vi "Control_Sensing_Sep.vi"() -> ()   [LabVIEW 2019]
uses:
  Control 1.ctl
  <vilib>/myRIO/Instrument Drivers/Onboard IO/I2C/typedefs/I2C User Configuration.ctl
  <vilib>/myRIO/Instrument Drivers/Onboard IO/I2C/typedefs/I2C Transfer Rate.ctl
  <vilib>/myRIO/Instrument Drivers/Onboard IO/I2C/typedefs/I2C Reference.ctl
  <vilib>/myRIO/Common/Instrument Driver Framework/Utilities/typedefs/myRIO Generic Hardware Reference.ctl
  <vilib>/myRIO/Common/Instrument Driver Framework/Utilities/typedefs/Hardware Version Enum.ctl
  <vilib>/myRIO/Common/Instrument Driver Framework/Utilities/typedefs/myRIO v1.0 Reference.ctl
  <vilib>/myRIO/Common/Instrument Driver Framework/Utilities/typedefs/Generic FPGA Reference.ctl
  <vilib>/myRIO/Common/Instrument Driver Framework/myRIO v1.0/I2C/typedefs/I2C Channels Enum.ctl
  <vilib>/myRIO/Instrument Drivers/Onboard IO/I2C/typedefs/I2C Configuration.ctl
  <vilib>/userDefined/High Color/nirio_resource_hc.ctl
  <vilib>/myRIO/Instrument Drivers/Onboard IO/DIO/typedefs/DIO Reference.ctl
  <vilib>/myRIO/Common/Instrument Driver Framework/myRIO v1.0/DIO/typedefs/DIO Channels List.ctl
  <vilib>/myRIO/Common/Instrument Driver Framework/myRIO v1.0/DIO/typedefs/DIO Channels Enum.ctl
  <vilib>/myRIO/Instrument Drivers/Onboard IO/AI/typedefs/AI Reference.ctl
  <vilib>/myRIO/Common/Instrument Driver Framework/myRIO v1.0/AI/typedefs/AI Channels List.ctl
  <vilib>/myRIO/Common/Instrument Driver Framework/myRIO v1.0/AI/typedefs/AI Channels Enum.ctl
  <vilib>/myRIO/Common/Instrument Driver Framework/Utilities/typedefs/Analog Scaling Constants List.ctl
  <vilib>/myRIO/Common/Instrument Driver Framework/Utilities/typedefs/Analog Scaling Constants.ctl
  <vilib>/myRIO/Instrument Drivers/Onboard IO/PWM/typedefs/PWM Reference.ctl
  <vilib>/myRIO/Common/Instrument Driver Framework/myRIO v1.0/PWM/typedefs/PWM Channels Enum.ctl
  <vilib>/myRIO/Instrument Drivers/Onboard IO/PWM/typedefs/PWM Configuration.ctl
  <vilib>/myRIO/Common/Instrument Driver Framework/Utilities/vis/Is FPGA Ref Available.vi
  <vilib>/myRIO/Common/Instrument Driver Framework/myRIO v1.0/I2C/vis/myRIO v1.1 Open I2C.vi
  <vilib>/myRIO/Instrument Drivers/Onboard IO/I2C/vis/Configure.vi
  <vilib>/myRIO/Instrument Drivers/Onboard IO/I2C/vis/Write.vi
  <vilib>/myRIO/Common/Instrument Driver Framework/myRIO v1.0/DIO/vis/myRIO v1.1 Open DIO.vi
  <vilib>/myRIO/Instrument Drivers/Onboard IO/DIO/vis/Write.vi
  <vilib>/myRIO/Common/Instrument Driver Framework/myRIO v1.0/AI/vis/myRIO v1.1 Open AI.vi
  <vilib>/myRIO/Instrument Drivers/Onboard IO/AI/vis/Read.vi
  <vilib>/myRIO/Common/Instrument Driver Framework/myRIO v1.0/PWM/vis/myRIO v1.1 Open PWM.vi
  <vilib>/myRIO/Instrument Drivers/Onboard IO/PWM/vis/Set Duty Cycle and Frequency.vi
  <vilib>/myRIO/Instrument Drivers/Onboard IO/I2C/vis/Write Read.vi
  <vilib>/myRIO/Common/Instrument Driver Framework/myRIO v1.0/UART/vis/myRIO v1.0 Close UART.vi
  <vilib>/myRIO/Common/Instrument Driver Framework/Utilities/vis/Validate Channels.vi
  <vilib>/myRIO/Common/Instrument Driver Framework/myRIO v1.0/I2C/vis/myRIO v1.0 Reserve I2C.vi
  <vilib>/myRIO/Common/Instrument Driver Framework/myRIO v1.0/DIO/vis/myRIO v1.0 Reserve DIO.vi
  <vilib>/myRIO/Common/Instrument Driver Framework/myRIO v1.0/AI/vis/myRIO v1.0 Reserve AI.vi
  <vilib>/myRIO/Common/Instrument Driver Framework/myRIO v1.0/PWM/vis/myRIO v1.0 Reserve PWM.vi
  <vilib>/myRIO/Common/Instrument Driver Framework/myRIO v1.0/I2C/vis/myRIO v1.0 Build MUX Configuration I2C.vi
  <vilib>/myRIO/Common/Instrument Driver Framework/myRIO v1.0/Resource Manager/vis/myRIO v1.0 Reserve Channel List.vi
  <vilib>/myRIO/Common/Instrument Driver Framework/myRIO v1.0/DIO/vis/myRIO v1.0 Build MUX Configuration DIO.vi
  <vilib>/myRIO/Common/Instrument Driver Framework/myRIO v1.0/AI/vis/myRIO v1.0 Build MUX Configuration AI.vi
  <vilib>/myRIO/Common/Instrument Driver Framework/myRIO v1.0/PWM/vis/myRIO v1.0 Build MUX Configuration PWM.vi
  <vilib>/myRIO/Common/Instrument Driver Framework/myRIO v1.0/Resource Manager/vis/myRIO v1.0 Create Configuration List.vi
  <vilib>/myRIO/Common/Instrument Driver Framework/myRIO v1.0/Resource Manager/vis/myRIO v1.0 Reserve Channel.vi
  <vilib>/myRIO/Common/Instrument Driver Framework/myRIO v1.0/Resource Manager/vis/myRIO v1.0 Unreserve Channel.vi
  <vilib>/myRIO/Common/Instrument Driver Framework/myRIO v1.0/Resource Manager/vis/myRIO v1.0 Build Mutex Name.vi
  <vilib>/imath/engines/lvmath2/RunTimeEngine/NodeEndStatement/NIMS_NodeEndStatement_Output.vi
  <instcachedir>/0/NIMS_NodeEndStatement_Output_53EC0D466D134D7ABD903AC30B43404B.lvgen/NIMS_NodeEndStatement_Output_53EC0D466D134D7ABD903AC30B43404B_000.vi
  <instcachedir>/0/NIMS_NodeEndStatement_Output_53EC0D466D134D7ABD903AC30B43404B.lvgen/NIMS_NodeEndStatement_Output_53EC0D466D134D7ABD903AC30B43404B_005.vi
  <vilib>/imath/engines/lvmath2/RunTimeEngine/ErrorHandling/NIMS_Finalize Error.vi
  <vilib>/imath/engines/lvmath2/RunTimeEngine/Managers/WorkSpace/UID Generator.vi
  <vilib>/imath/engines/lvmath2/RunTimeEngine/RunTimeType/NIMS_RunTimeType_From StrictType (excl LVString).vi
  <instcachedir>/0/NIMS_RunTimeType_From StrictType (excl LVString)_D8AFBA86A94845AAA577C895450664BD.lvgen/NIMS_RunTimeType_From StrictType (excl LVString)_D8AFBA86A94845AAA577C895450664BD_000.vi
  <vilib>/imath/engines/lvmath2/RunTimeEngine/LocalVariableDefStatement/MC_LocalVariableDefStatement_Display.vi
  <vilib>/imath/engines/lvmath2/RunTimeEngine/RangeToken/NIMS_Range.vi
  <instcachedir>/0/NIMS_Range_FADF6ADDA3E145BB934C8BD4C7DAAB97.lvgen/NIMS_Range_FADF6ADDA3E145BB934C8BD4C7DAAB97_000.vi
  <vilib>/imathl/engines/lvmath/Functions/Error Handling/Create Error.vi
  <vilib>/imath/engines/lvmath2/RunTimeEngine/BuiltInFunctions/length/NIMS_length(GV).vi
  <instcachedir>/0/NIMS_length(GV)_08A3D13377FD4E4B96F5795FBF3698FA.lvgen/NIMS_length(GV)_08A3D13377FD4E4B96F5795FBF3698FA_000.vi
  <vilib>/imath/engines/lvmath2/RunTimeEngine/BuiltInFunctions/ones/NIMS_V=ones(I32,I32).vi
  <vilib>/imath/engines/lvmath2/RunTimeEngine/Managers/SymbolTable/Clear UID.vi
  <vilib>/imath/engines/lvmath2/RunTimeEngine/BuiltInFunctions/diag/NIMS_diag.vi
  <instcachedir>/0/NIMS_diag_DCAB8C8FDAF64F9E84492BB524435AA9.lvgen/NIMS_diag_DCAB8C8FDAF64F9E84492BB524435AA9_003.vi
  <vilib>/imath/engines/lvmath2/RunTimeEngine/BuiltInFunctions/mirrorh/NIMS_mirrorh(GM).vi
  <instcachedir>/0/NIMS_mirrorh(GM)_A650AD0D730A4A8EBE251B4C5C7CA115.lvgen/NIMS_mirrorh(GM)_A650AD0D730A4A8EBE251B4C5C7CA115_004.vi
  <vilib>/imath/engines/lvmath2/RunTimeEngine/RowToken/NIMS_RowToken_M_M.vi
  <instcachedir>/0/NIMS_RowToken_M_M_21FE36D058524603B8B587AC30FD72C2.lvgen/NIMS_RowToken_M_M_21FE36D058524603B8B587AC30FD72C2_005.vi
  <vilib>/imath/engines/lvmath2/RunTimeEngine/ErrorHandling/NIMS_Create Error From Enums.vi
  <instcachedir>/0/NIMS_NodeEndStatement_Output_53EC0D466D134D7ABD903AC30B43404B.lvgen/NIMS_NodeEndStatement_Output_53EC0D466D134D7ABD903AC30B43404B_002.vi
  <instcachedir>/0/NIMS_NodeEndStatement_Output_53EC0D466D134D7ABD903AC30B43404B.lvgen/NIMS_NodeEndStatement_Output_53EC0D466D134D7ABD903AC30B43404B_010.vi
  <vilib>/Utility/VariantDataType/GetNumericInfo.vi
  <vilib>/Utility/error.llb/Error Cluster From Error Code.vi
  <vilib>/myRIO/Common/Instrument Driver Framework/myRIO v1.0/myRIO v1.1 Open.vi
  <vilib>/myRIO/Common/Instrument Driver Framework/Utilities/vis/IO Manager.vi
  <vilib>/myRIO/Common/Instrument Driver Framework/Utilities/vis/Configuration Manager.vi
  <vilib>/myRIO/Common/Instrument Driver Framework/myRIO v1.0/Resource Manager/vis/myRIO v1.0 Configure IO.vi
  <vilib>/myRIO/Common/Instrument Driver Framework/myRIO v1.0/myRIO v1.0 Close.vi
  <vilib>/myRIO/Common/Instrument Driver Framework/myRIO v1.0/I2C/vis/myRIO v1.0 Configure I2C.vi
  <vilib>/myRIO/Common/Instrument Driver Framework/myRIO v1.0/I2C/vis/myRIO v1.0 Write I2C.vi
  <vilib>/myRIO/Common/Instrument Driver Framework/myRIO v1.0/DIO/vis/myRIO v1.0 Write DIO.vi
  <vilib>/myRIO/Common/Instrument Driver Framework/myRIO v1.0/AI/vis/myRIO v1.0 Get Scaling Constants AI.vi
  <vilib>/myRIO/Common/Instrument Driver Framework/myRIO v1.0/AI/vis/myRIO v1.0 Read AI.vi
  <vilib>/myRIO/Common/Instrument Driver Framework/myRIO v1.0/PWM/vis/myRIO v1.0 Write PWM.vi
  <vilib>/myRIO/Common/Instrument Driver Framework/myRIO v1.0/I2C/vis/myRIO v1.0 Read I2C.vi
  LabVIEW Data/MathScriptVIs/MCStatic_41946317732_fa5be5f0b8b257016d1ff6cc8f1b5180.vi
  <instcachedir>/0/MCStatic_41946317732_fa5be5f0b8b257016d1ff6cc8f1b5180_9A0A86F2D3274CCBAD522B545B9D9F0A.lvgen/MCStatic_41946317732_fa5be5f0b8b257016d1ff6cc8f1b5180_9A0A86F2D3274CCBAD522B545B9D9F0A_001.vi
  <vilib>/imath/engines/lvmath2/RunTimeEngine/ArithmeticOperatorToken/NIMS_ArithmeticOperator_multmx.vi
  <instcachedir>/0/NIMS_ArithmeticOperator_multmx_77F1D2D6F4D94BA7A97C4E7185C02392.lvgen/NIMS_ArithmeticOperator_multmx_77F1D2D6F4D94BA7A97C4E7185C02392_003.vi
  <instcachedir>/0/NIMS_diag_DCAB8C8FDAF64F9E84492BB524435AA9.lvgen/NIMS_diag_DCAB8C8FDAF64F9E84492BB524435AA9_002.vi
  <vilib>/imath/engines/lvmath2/RunTimeEngine/BuiltInFunctions/max/1 input/NIMS_max(CM).vi
  <instcachedir>/0/NIMS_max(CM)_ECFF9CEF2CF74B92B05BC258ECD38873.lvgen/NIMS_max(CM)_ECFF9CEF2CF74B92B05BC258ECD38873_000.vi
  <vilib>/imath/engines/lvmath/Functions/Error Handling/MergeErrorsWrapper.vi
  <vilib>/imath/engines/lvmath2/RunTimeEngine/CommandStatement/MC_CommandStatement_break.vi
  LabVIEW Data/MathScriptVIs/MCStatic_41946317732_32a02ef49a6087299864d0ca1f279a51.vi
  <instcachedir>/0/MCStatic_41946317732_32a02ef49a6087299864d0ca1f279a51_171346ACDDCF4ECDA237C5453963259D.lvgen/MCStatic_41946317732_32a02ef49a6087299864d0ca1f279a51_171346ACDDCF4ECDA237C5453963259D_000.vi
  <vilib>/imath/engines/lvmath2/RunTimeEngine/ArithmeticOperatorToken/NIMS_ArithmeticOperator_minus.vi
  <instcachedir>/0/NIMS_ArithmeticOperator_minus_12BFF9710EA5430A9EE87C5BC3F65186.lvgen/NIMS_ArithmeticOperator_minus_12BFF9710EA5430A9EE87C5BC3F65186_009.vi
  <vilib>/imath/engines/lvmath2/RunTimeEngine/BuiltInFunctions/norm/NIMS_norm(GM,DBL).vi
  <instcachedir>/0/NIMS_norm(GM,DBL)_8BCB088F207E48DF95CF5C1DC502F84D.lvgen/NIMS_norm(GM,DBL)_8BCB088F207E48DF95CF5C1DC502F84D_001.vi
  <vilib>/imath/engines/lvmath2/RunTimeEngine/BuiltInFunctions/abs/NIMS_abs(signed).vi
  <instcachedir>/0/NIMS_abs(signed)_C4FCB8E6058B49B797C7C8D53CA5F6EC.lvgen/NIMS_abs(signed)_C4FCB8E6058B49B797C7C8D53CA5F6EC_003.vi
  <vilib>/imath/engines/lvmath2/RunTimeEngine/BuiltInFunctions/max/1 input/NIMS_max(RM).vi
  <instcachedir>/0/NIMS_max(RM)_0B4294876EE440609D638D7C5C6E788E.lvgen/NIMS_max(RM)_0B4294876EE440609D638D7C5C6E788E_000.vi
  <vilib>/imath/engines/lvmath2/RunTimeSupport/NIMS_Get Scalar_w Error.vi
  <instcachedir>/0/NIMS_Get Scalar_w Error_90FA09EFB1C84794B43793796939E0E3.lvgen/NIMS_Get Scalar_w Error_90FA09EFB1C84794B43793796939E0E3_010.vi
  <vilib>/imath/engines/lvmath2/RunTimeEngine/BuiltInFunctions/eye/NIMS_M=eye(I32).vi
  <instcachedir>/0/NIMS_ArithmeticOperator_multmx_77F1D2D6F4D94BA7A97C4E7185C02392.lvgen/NIMS_ArithmeticOperator_multmx_77F1D2D6F4D94BA7A97C4E7185C02392_006.vi
  <vilib>/imath/engines/lvmath2/RunTimeEngine/ArithmeticOperatorToken/NIMS_ArithmeticOperator_plus.vi
  <instcachedir>/0/NIMS_ArithmeticOperator_plus_5C9385B0197D46E2B844C41E02F9EC39.lvgen/NIMS_ArithmeticOperator_plus_5C9385B0197D46E2B844C41E02F9EC39_002.vi
  <vilib>/imath/engines/lvmath2/RunTimeEngine/ArithmeticOperatorToken/NIMS_ArithmeticOperator_leftdivmx(C,C).vi
  <instcachedir>/0/NIMS_ArithmeticOperator_leftdivmx(C,C)_FFA86DC98B994D28AA7593516F1DAFDA.lvgen/NIMS_ArithmeticOperator_leftdivmx(C,C)_FFA86DC98B994D28AA7593516F1DAFDA_000.vi
  <vilib>/imath/engines/lvmath2/RunTimeEngine/ArithmeticOperatorToken/NIMS_ArithmeticOperator_rightdiv.vi
  <instcachedir>/0/NIMS_ArithmeticOperator_rightdiv_23AAA10E4B1E4564B1AF1956090A34B0.lvgen/NIMS_ArithmeticOperator_rightdiv_23AAA10E4B1E4564B1AF1956090A34B0_004.vi
  <instcachedir>/0/NIMS_ArithmeticOperator_minus_12BFF9710EA5430A9EE87C5BC3F65186.lvgen/NIMS_ArithmeticOperator_minus_12BFF9710EA5430A9EE87C5BC3F65186_008.vi
  <vilib>/imath/engines/lvmath2/RunTimeEngine/ArithmeticOperatorToken/NIMS_ArithmeticOperator_rightdivmx(C,C).vi
  <instcachedir>/0/NIMS_ArithmeticOperator_rightdivmx(C,C)_4C9834AF73264B85B2EC0ABB36B07CCF.lvgen/NIMS_ArithmeticOperator_rightdivmx(C,C)_4C9834AF73264B85B2EC0ABB36B07CCF_000.vi
  <vilib>/imath/engines/lvmath2/RunTimeEngine/ArithmeticOperatorToken/NIMS_ArithmeticOperator_powermx(M,M).vi
  <vilib>/imath/engines/lvmath2/RunTimeEngine/BuiltInFunctions/max/2 inputs/NIMS_max(CG,CG)-no size check.vi
  <instcachedir>/0/NIMS_max(CG,CG)-no size check_0D8807EB624448B1961BA94FD6C7666D.lvgen/NIMS_max(CG,CG)-no size check_0D8807EB624448B1961BA94FD6C7666D_000.vi
  <instcachedir>/0/MCStatic_41946317732_fa5be5f0b8b257016d1ff6cc8f1b5180_9A0A86F2D3274CCBAD522B545B9D9F0A.lvgen/MCStatic_41946317732_fa5be5f0b8b257016d1ff6cc8f1b5180_9A0A86F2D3274CCBAD522B545B9D9F0A_000.vi
  <vilib>/imath/engines/lvmath2/RunTimeEngine/CommandStatement/NIMS_CommandStatement_MaskErr.vi
  <vilib>/imath/engines/lvmath2/RunTimeEngine/NodeEndStatement/NIMS_NodeEndStatement_Get Vector.vi
  <instcachedir>/0/NIMS_NodeEndStatement_Get Vector_92F29E6578CC4FEABDAC0B727A70E862.lvgen/NIMS_NodeEndStatement_Get Vector_92F29E6578CC4FEABDAC0B727A70E862_003.vi
  LabVIEW Data/MathScriptVIs/MCStatic_41946317732_98f405ff8d5ce23d3fe31c5b01ac1feb.vi
  <instcachedir>/0/MCStatic_41946317732_98f405ff8d5ce23d3fe31c5b01ac1feb_64A766A8D52149F492EA82AFF1B0937C.lvgen/MCStatic_41946317732_98f405ff8d5ce23d3fe31c5b01ac1feb_64A766A8D52149F492EA82AFF1B0937C_001.vi
  LabVIEW Data/MathScriptVIs/MCStatic_41946317732_f51fcaa409b1ee3974faba1f5ada3bee.vi
  <instcachedir>/0/MCStatic_41946317732_f51fcaa409b1ee3974faba1f5ada3bee_1946984F0DF54B0185DA9AD754108A45.lvgen/MCStatic_41946317732_f51fcaa409b1ee3974faba1f5ada3bee_1946984F0DF54B0185DA9AD754108A45_000.vi
  <instcachedir>/0/MCStatic_41946317732_98f405ff8d5ce23d3fe31c5b01ac1feb_64A766A8D52149F492EA82AFF1B0937C.lvgen/MCStatic_41946317732_98f405ff8d5ce23d3fe31c5b01ac1feb_64A766A8D52149F492EA82AFF1B0937C_000.vi
  <vilib>/myRIO/Common/Instrument Driver Framework/Utilities/vis/FPGA Ref Manager.vi
  <vilib>/myRIO/Common/Instrument Driver Framework/myRIO v1.0/myRIO v1.0 Reset FPGA.vi
  <vilib>/myRIO/Common/Instrument Driver Framework/myRIO v1.0/IRQ/vis/myRIO v1.0 IRQ Info FGV.vi
  <vilib>/myRIO/Common/Instrument Driver Framework/myRIO v1.0/IRQ/vis/myRIO v1.0 Timer IRQ Info FGV.vi
  <vilib>/myRIO/Common/Instrument Driver Framework/myRIO v1.0/IRQ/vis/myRIO v1.0 ISR Agent.vi
  <vilib>/myRIO/Instrument Drivers/Utilities/vis/Reset Index.vi
  <vilib>/myRIO/Common/Instrument Driver Framework/myRIO v1.0/Resource Manager/vis/myRIO v1.0 Block Write Resource Manager.vi
  <vilib>/myRIO/Express VI/Onboard IO/I2C/I2C Express VI.xnode
  <vilib>/myRIO/Instrument Drivers/Onboard IO/I2C/vis/myRIO I2C Open.xnode
  <vilib>/myRIO/Express VI/Onboard IO/DO/DO Express VI.xnode
  <vilib>/myRIO/Instrument Drivers/Onboard IO/DIO/vis/myRIO DIO Open.xnode
  <vilib>/myRIO/Express VI/Onboard IO/AI/AI Express VI.xnode
  <vilib>/myRIO/Instrument Drivers/Onboard IO/AI/vis/myRIO AI Open.xnode
  <vilib>/myRIO/Express VI/Onboard IO/PWM/PWM Express VI.xnode
  <vilib>/myRIO/Instrument Drivers/Onboard IO/PWM/vis/myRIO PWM Open.xnode
  magnetic_sensing-main/Analytic_Jacobian_Mag_cir_array_noM.m
  magnetic_sensing-main/PM_forward_field_noM.m
  magnetic_sensing-main/Analytic_Jacobian_Mag_cir_array_test.m
  magnetic_sensing-main/PM_forward_field.m
  <vilib>/myRIO/Instrument Drivers/Onboard IO/I2C/I2C.lvlib
  <vilib>/myRIO/Instrument Drivers/Utilities/Utilities.lvlib
  <vilib>/myRIO/Instrument Drivers/Onboard IO/PWM/PWM.lvlib
  <vilib>/myRIO/Instrument Drivers/Onboard IO/DIO/DIO.lvlib
  <vilib>/myRIO/Instrument Drivers/Onboard IO/AI/AI.lvlib
  <vilib>/imath/engines/lvmath2/RunTimeEngine/Managers/SymbolTable/NIMS_WorkSpace.lvlib
  <instcachedir>/0/MCStatic_41946317732_32a02ef49a6087299864d0ca1f279a51_171346ACDDCF4ECDA237C5453963259D.lvgen/MCStatic_41946317732_32a02ef49a6087299864d0ca1f279a51_171346ACDDCF4ECDA237C5453963259D_001.vi
  <instcachedir>/0/MCStatic_41946317732_f51fcaa409b1ee3974faba1f5ada3bee_1946984F0DF54B0185DA9AD754108A45.lvgen/MCStatic_41946317732_f51fcaa409b1ee3974faba1f5ada3bee_1946984F0DF54B0185DA9AD754108A45_001.vi
panel:
  in  "Reset Feeding":bool
  in  "Reset Actuation":bool
  in  "Enum":T1(ring)
  in  "Steer Gain (2.3)":dbl
  out "feed displacement":dbl
  out "Feed Encoder 2":dbl(graph)
  out "Degree Angle":dbl
  out "y act":dbl
  out "X act":dbl
  out "delta x":dbl
  out "delta Y":dbl
  out "Duty Ratio":dbl
  out "Steer Encoder":dbl(graph)
  out "Sensing time":u32
  in  "M (0.0395266)":dbl
  in  "Update M in realtime?":bool
  in  "Clear plot?":bool
  out "pm_hat_opt":dbl[](array[numeric])
  in  "stop":bool
  in  "Actuation on?":bool
  in  "Action Mode":T2=enum."Sensing"
  out "XY Graph":cluster{dbl[], dbl[]}[](graph)
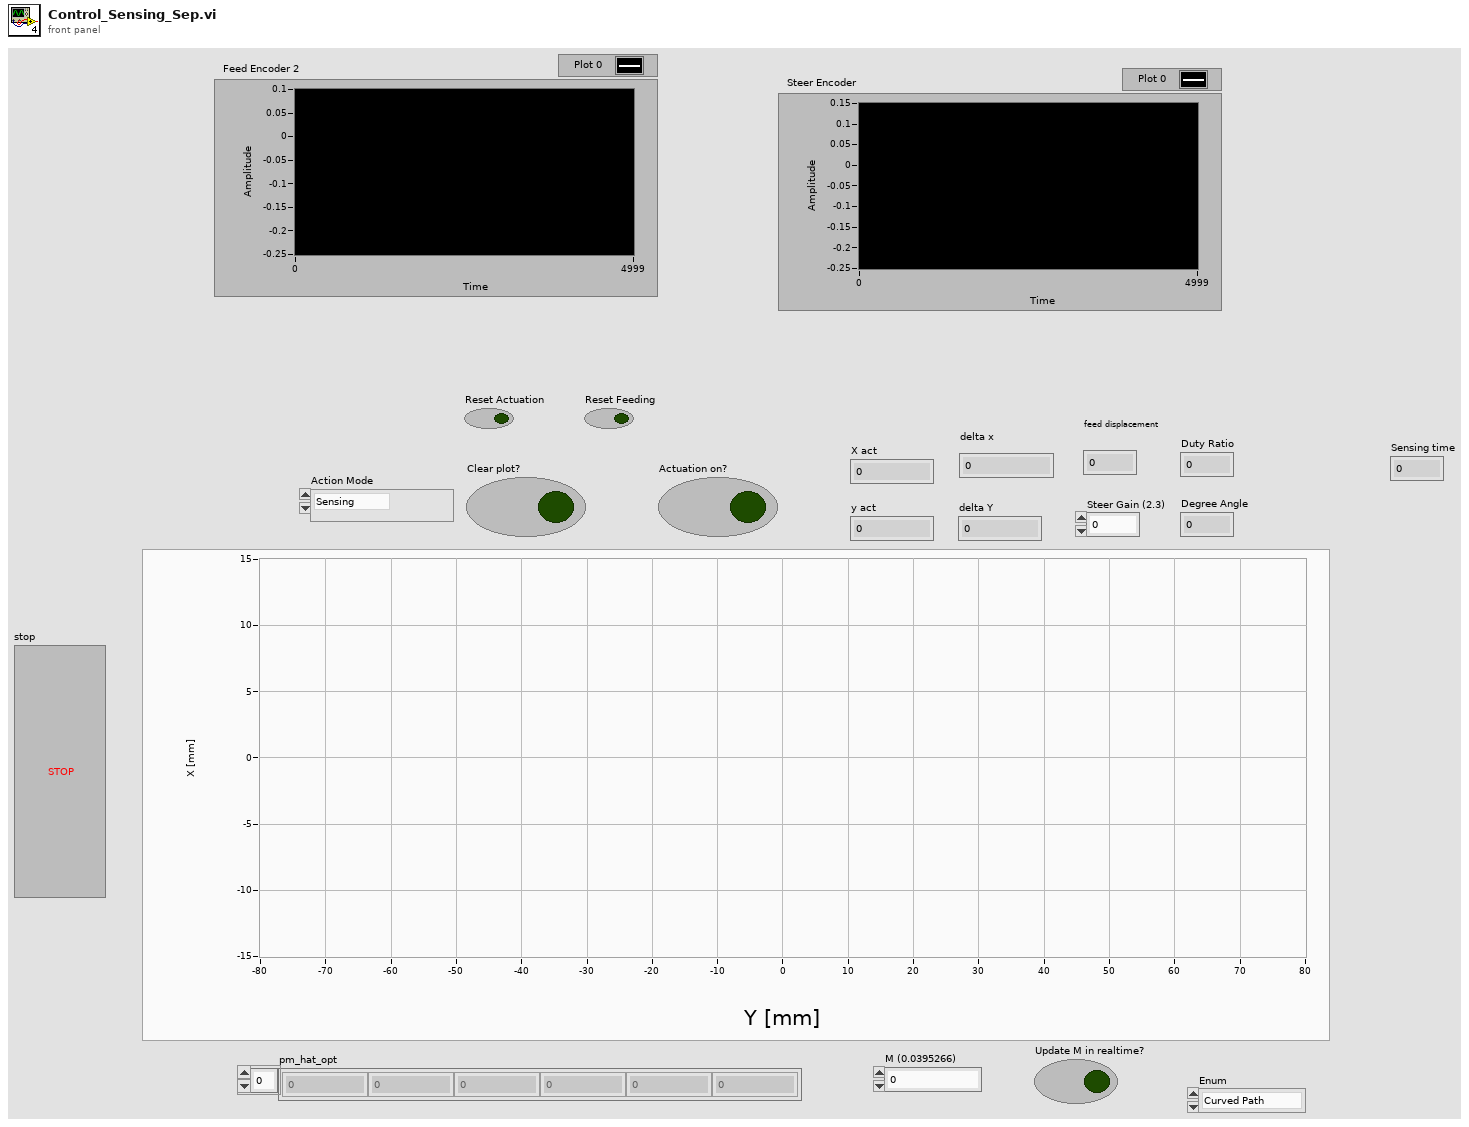
[diagram p1: front panel]
types:
  T1 = enum16{"Curved Path", "Bifurcation", "Branch off"}
  T2 = typedef "Control 1.ctl" = enum16{"Actuation", "Waiting", "Sensing"}
  T3 = typedef "I2C.lvlib/I2C Reference.ctl" = cluster{"myRIO Reference":T4, "I2C Channels Enum":T8, "I2C Configuration":T9}
  T4 = typedef "myRIO Generic Hardware Reference.ctl" = cluster{"myRIO Model":T5, "myRIO Hardware Reference":T6}
  T5 = typedef "Hardware Version Enum.ctl" = enum16{"Unknown", "myRIO-1900", "myRIO-1950", "roboRIO", "NI ELVIS RIO CM", "ELVIS III"}
  T6 = typedef "myRIO v1.0 Reference.ctl" = cluster{"Generic FPGA Reference":T7, "Allow multiple opens":bool}
  T7 = typedef "Generic FPGA Reference.ctl" = refnum<k20>
  T8 = typedef "I2C Channels Enum.ctl" = enum16{"Not Connected", "A/I2C", "B/I2C", "I2C/I2C"}
  T9 = typedef "I2C.lvlib/I2C Configuration.ctl" = cluster{"I2C Transfer Rate":T10}
  T10 = typedef "I2C.lvlib/I2C Transfer Rate.ctl" = enum16{"Standard mode (100 kbps)", "Fast mode (400 kbps)"}
  T11 = typedef "I2C.lvlib/I2C User Configuration.ctl" = cluster{"I2C Transfer Rate":T10}
  T12 = typedef "nirio_resource_hc.ctl" = tag
  T13 = typedef "DIO.lvlib/DIO Reference.ctl" = cluster{"myRIO Reference":T4, "DIO Channels List":T14}
  T14 = typedef "DIO Channels List.ctl" = T15[]
  T15 = typedef "DIO Channels Enum.ctl" = enum16{"Not Connected", "C/DIO0", "C/DIO1", "C/DIO2", "C/DIO3", "C/DIO4", "C/DIO5", "C/DIO6", "C/DIO7", "A/DIO0", "A/DIO1", "A/DIO2", "A/DIO3", "A/DIO4", "A/DIO5", "A/DIO6", "A/DIO7", "A/DIO8", "A/DIO9", "A/DIO10", "A/DIO11", "A/DIO12", "A/DIO13", "A/DIO14", "A/DIO15", "A/DIO16", "A/DIO17", "A/DIO18", "A/DIO19", "B/DIO0", "B/DIO1", "B/DIO2", "B/DIO3", "B/DIO4", "B/DIO5", "B/DIO6", "B/DIO7", "B/DIO8", "B/DIO9", "B/DIO10", "B/DIO11", "B/DIO12", "B/DIO13", "B/DIO14", "B/DIO15", "B/DIO16", "B/DIO17", "B/DIO18", "B/DIO19", "LED0", "LED1", "LED2", "LED3", "Button0", "DIO/DIO0", "DIO/DIO1", "DIO/DIO2", "DIO/DIO3", "DIO/DIO4", "DIO/DIO5", "DIO/DIO6", "DIO/DIO7", "DIO/DIO8", "DIO/DIO9", "SPI/CS0", "SPI/CS1", "SPI/CS2", "SPI/CS3", "LED RADIO (Green)", "LED RADIO (Red)", "LED COMM (Green)", "LED COMM (Red)", "LED MODE (Green)", "LED MODE (Red)"}
  T16 = typedef "AI.lvlib/AI Reference.ctl" = cluster{"myRIO Reference":T4, "AI Channels List":T17, "AI Scaling Constants List":T19}
  T17 = typedef "AI Channels List.ctl" = T18[]
  T18 = typedef "AI Channels Enum.ctl" = enum16{"Not Connected", "AudioIn/Left", "AudioIn/Right", "C/AI0", "C/AI1", "A/AI0", "A/AI1", "A/AI2", "A/AI3", "A/AI4", "A/AI5", "A/AI6", "A/AI7", "B/AI0", "B/AI1", "B/AI2", "B/AI3", "B/AI4", "B/AI5", "B/AI6", "B/AI7", "AI/AI0", "AI/AI1", "AI/AI2", "AI/AI3", "A/AI0 (DIFF)", "A/AI1 (DIFF)", "A/AI2 (DIFF)", "A/AI3 (DIFF)", "B/AI0 (DIFF)", "B/AI1 (DIFF)", "B/AI2 (DIFF)", "B/AI3 (DIFF)"}
  T19 = typedef "Analog Scaling Constants List.ctl" = T20[]
  T20 = typedef "Analog Scaling Constants.ctl" = cluster{"LSB Weight (Volts)":dbl, "Offset (Volts)":dbl, "Signed?":bool}
  T21 = typedef "PWM.lvlib/PWM Reference.ctl" = cluster{"myRIO Reference":T4, "PWM Channels Enum":T22, "PWM Configuration":T23}
  T22 = typedef "PWM Channels Enum.ctl" = enum16{"Not Connected", "C/PWM0", "C/PWM1", "A/PWM0", "A/PWM1", "A/PWM2", "A/PWM3", "A/PWM4", "A/PWM5", "A/PWM6", "A/PWM7", "A/PWM8", "A/PWM9", "A/PWM10", "A/PWM11", "A/PWM12", "A/PWM13", "A/PWM14", "A/PWM15", "A/PWM16", "A/PWM17", "A/PWM18", "A/PWM19", "B/PWM0", "B/PWM1", "B/PWM2", "B/PWM3", "B/PWM4", "B/PWM5", "B/PWM6", "B/PWM7", "B/PWM8", "B/PWM9", "B/PWM10", "B/PWM11", "B/PWM12", "B/PWM13", "B/PWM14", "B/PWM15", "B/PWM16", "B/PWM17", "B/PWM18", "B/PWM19", "PWM/PWM0", "PWM/PWM1", "PWM/PWM2", "PWM/PWM3", "PWM/PWM4", "PWM/PWM5", "PWM/PWM6", "PWM/PWM7", "PWM/PWM8", "PWM/PWM9"}
  T23 = typedef "PWM.lvlib/PWM Configuration.ctl" = cluster{"Frequency":dbl, "Duty Cycle":dbl}
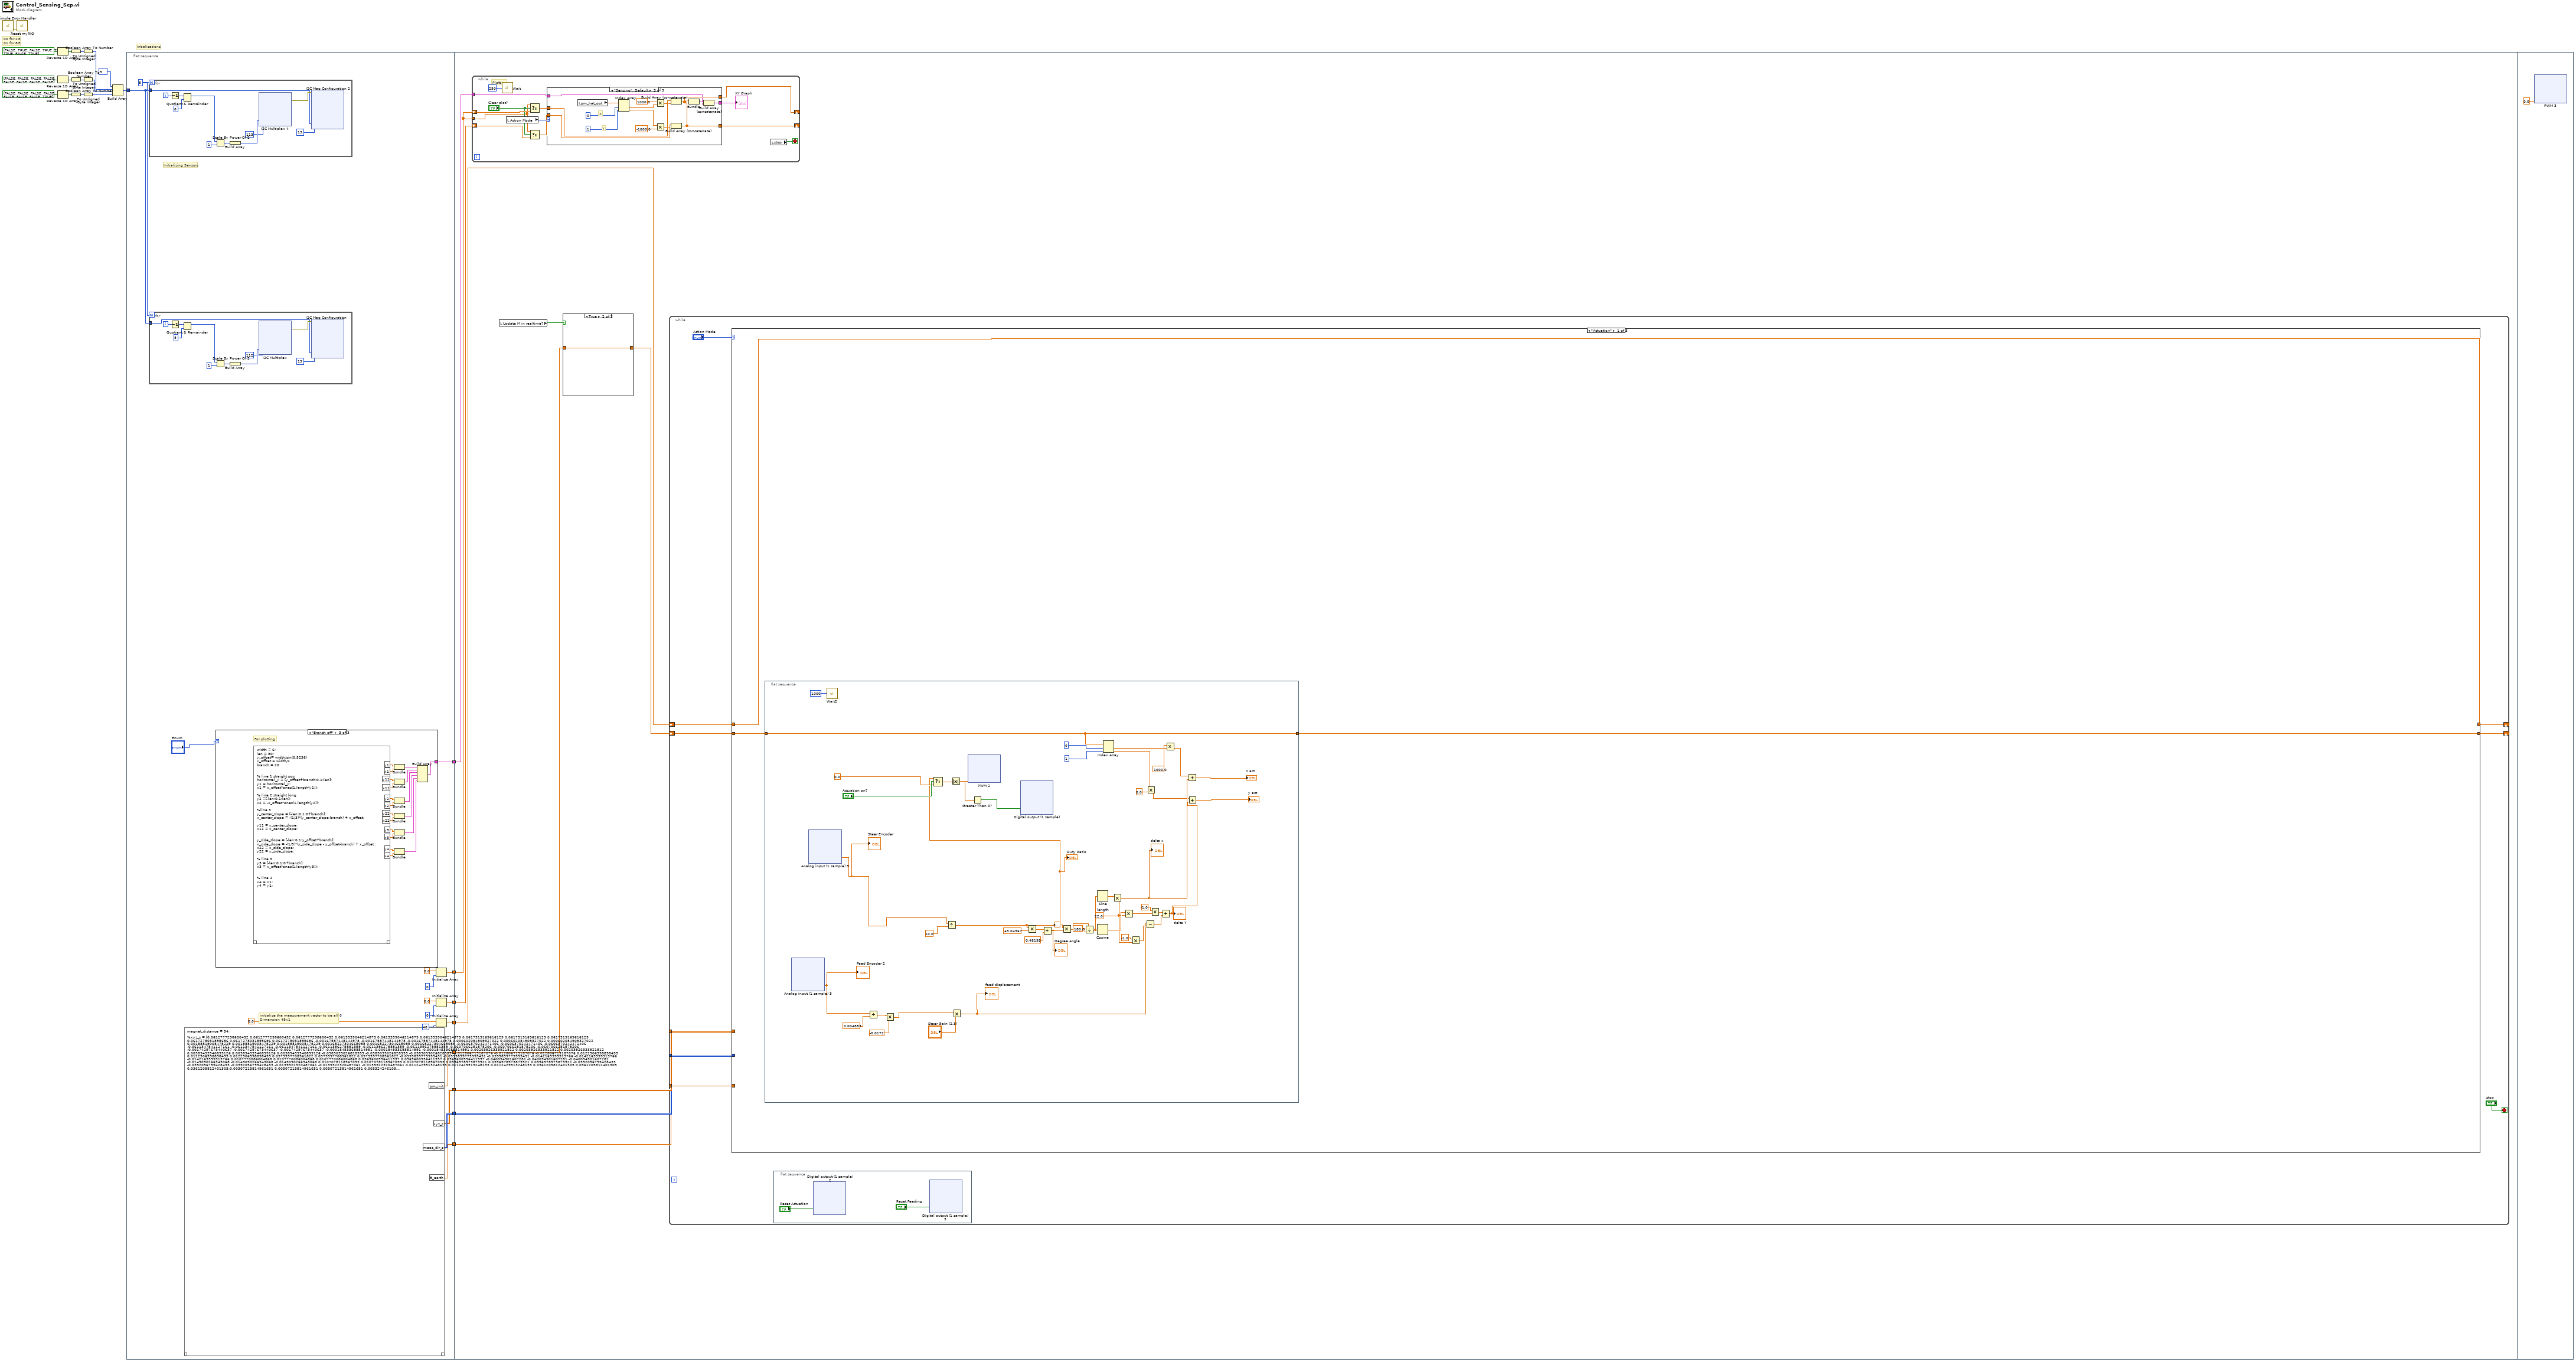
[diagram p0: block diagram]
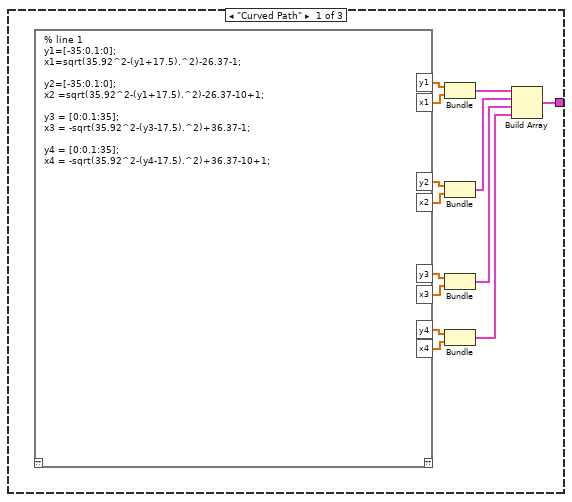
[diagram p2: hidden frame]
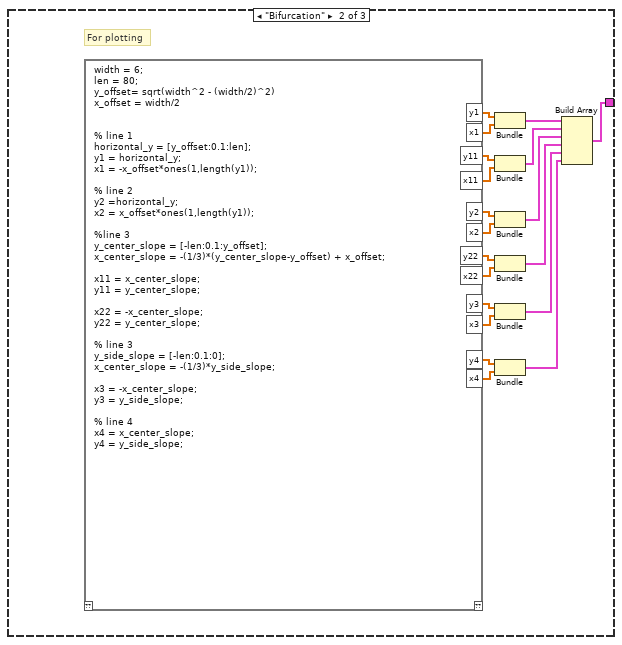
[diagram p3: hidden frame]
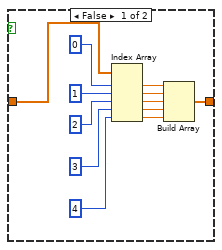
[diagram p4: hidden frame]
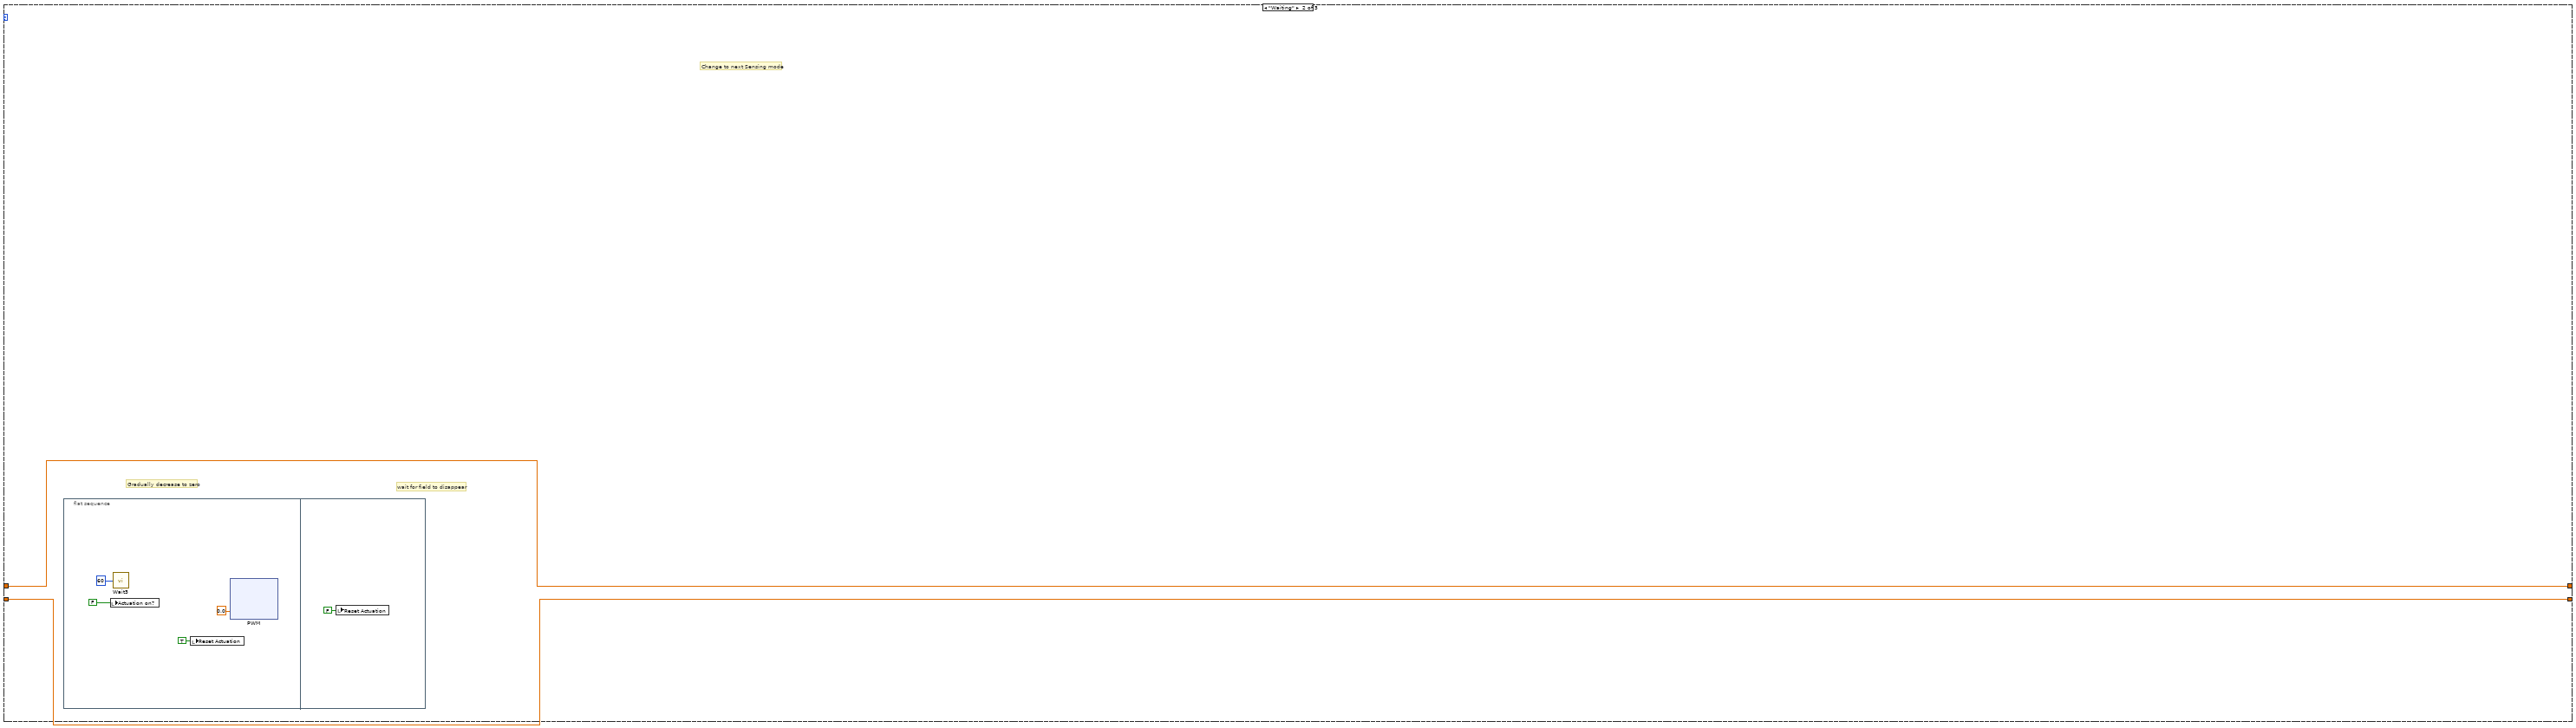
[diagram p5: hidden frame]
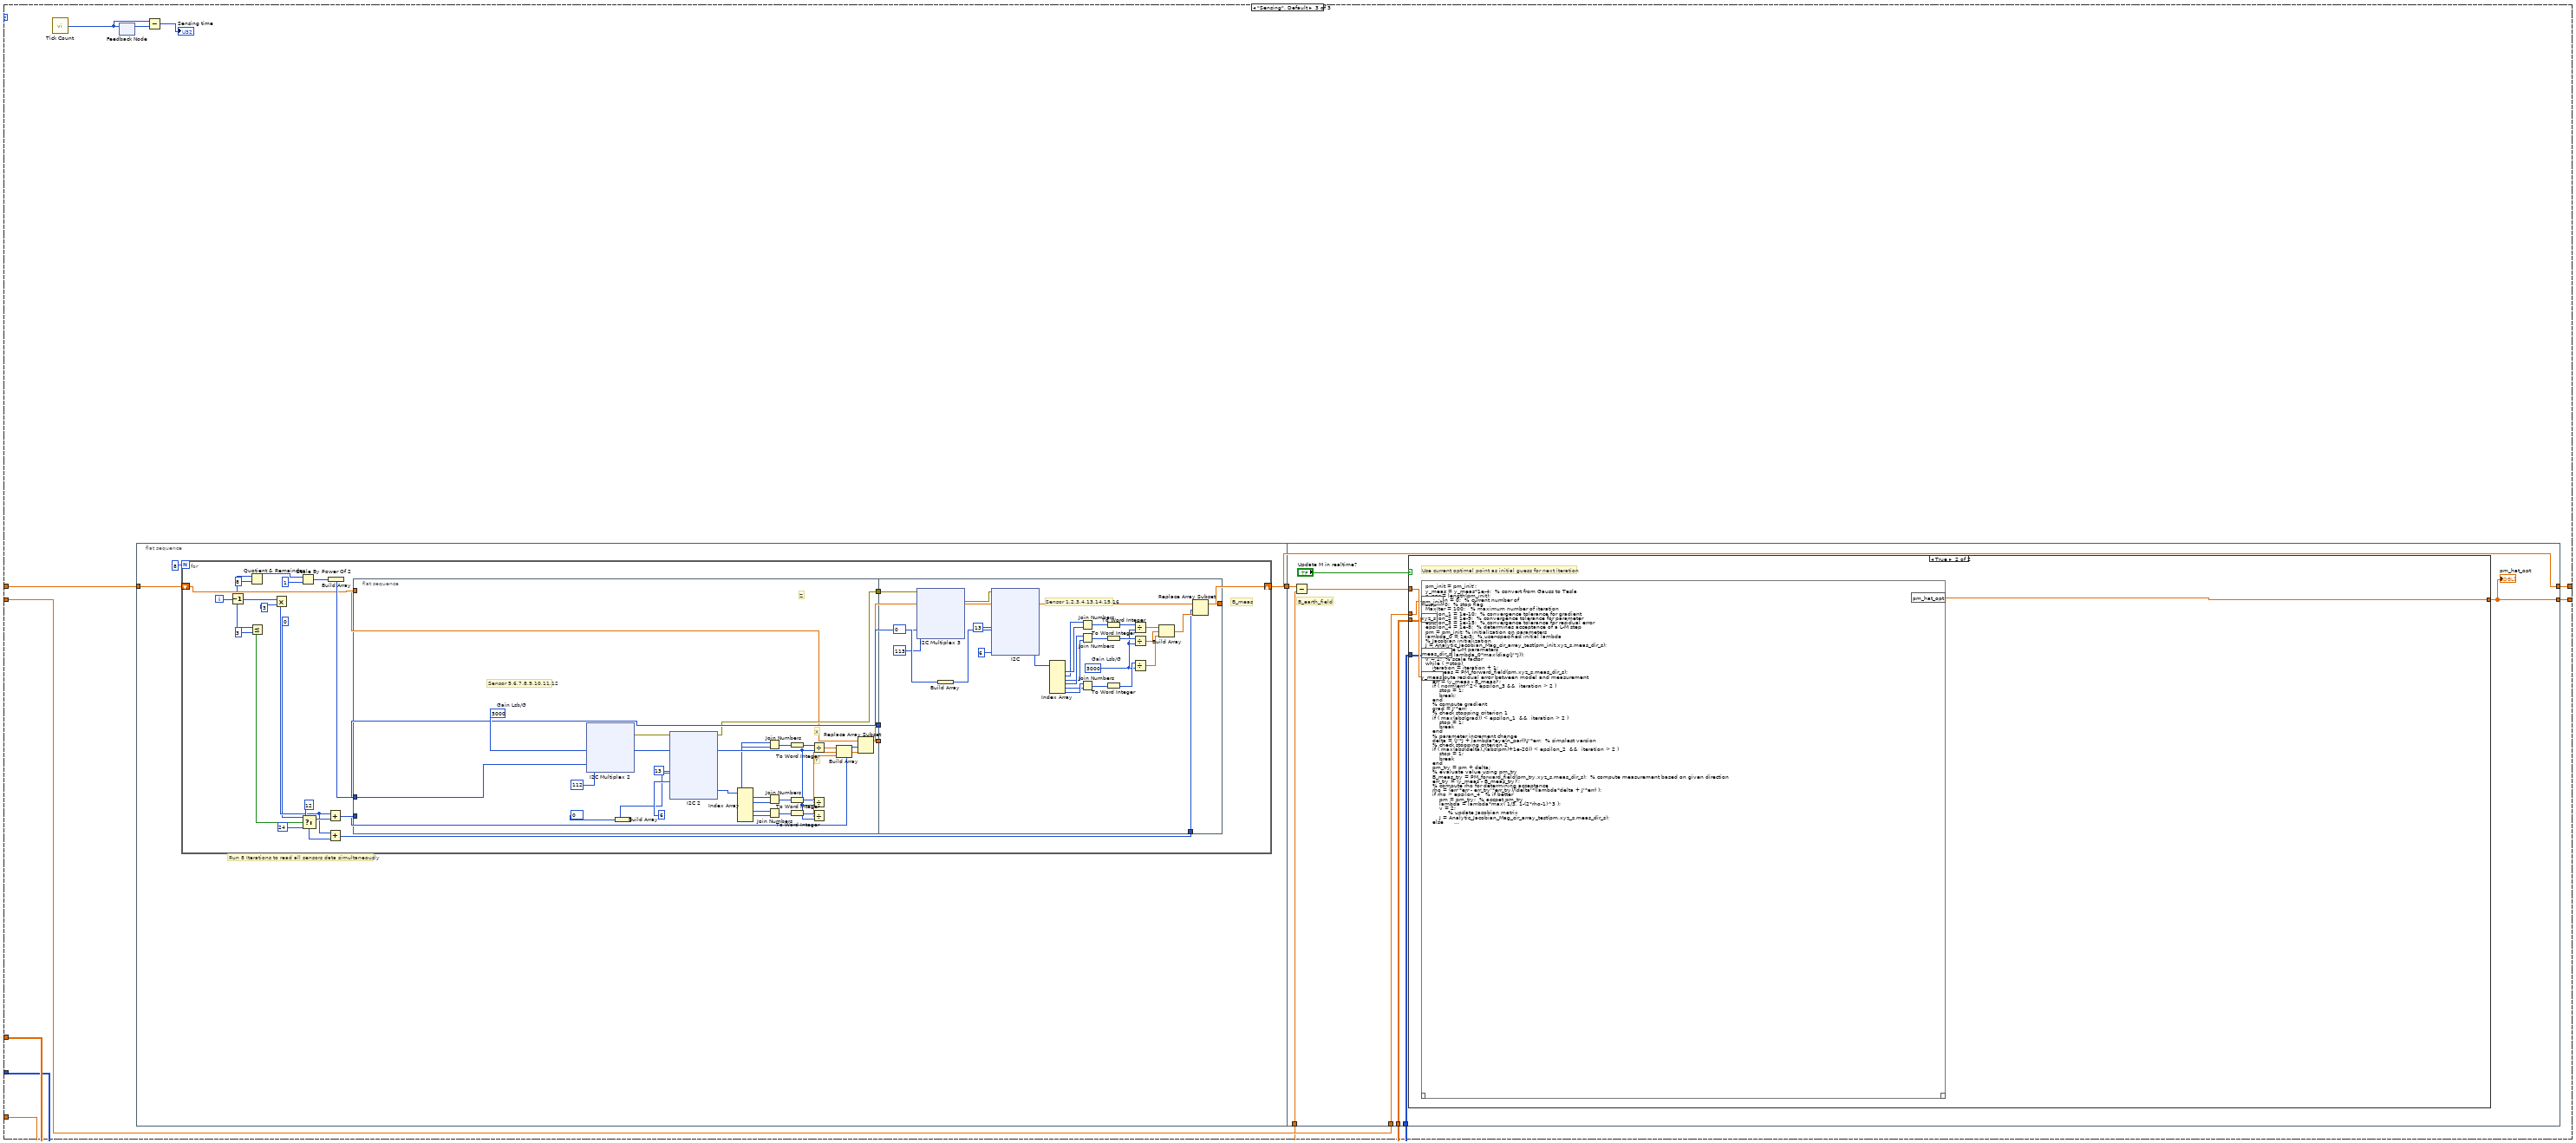
[diagram p6: hidden frame]
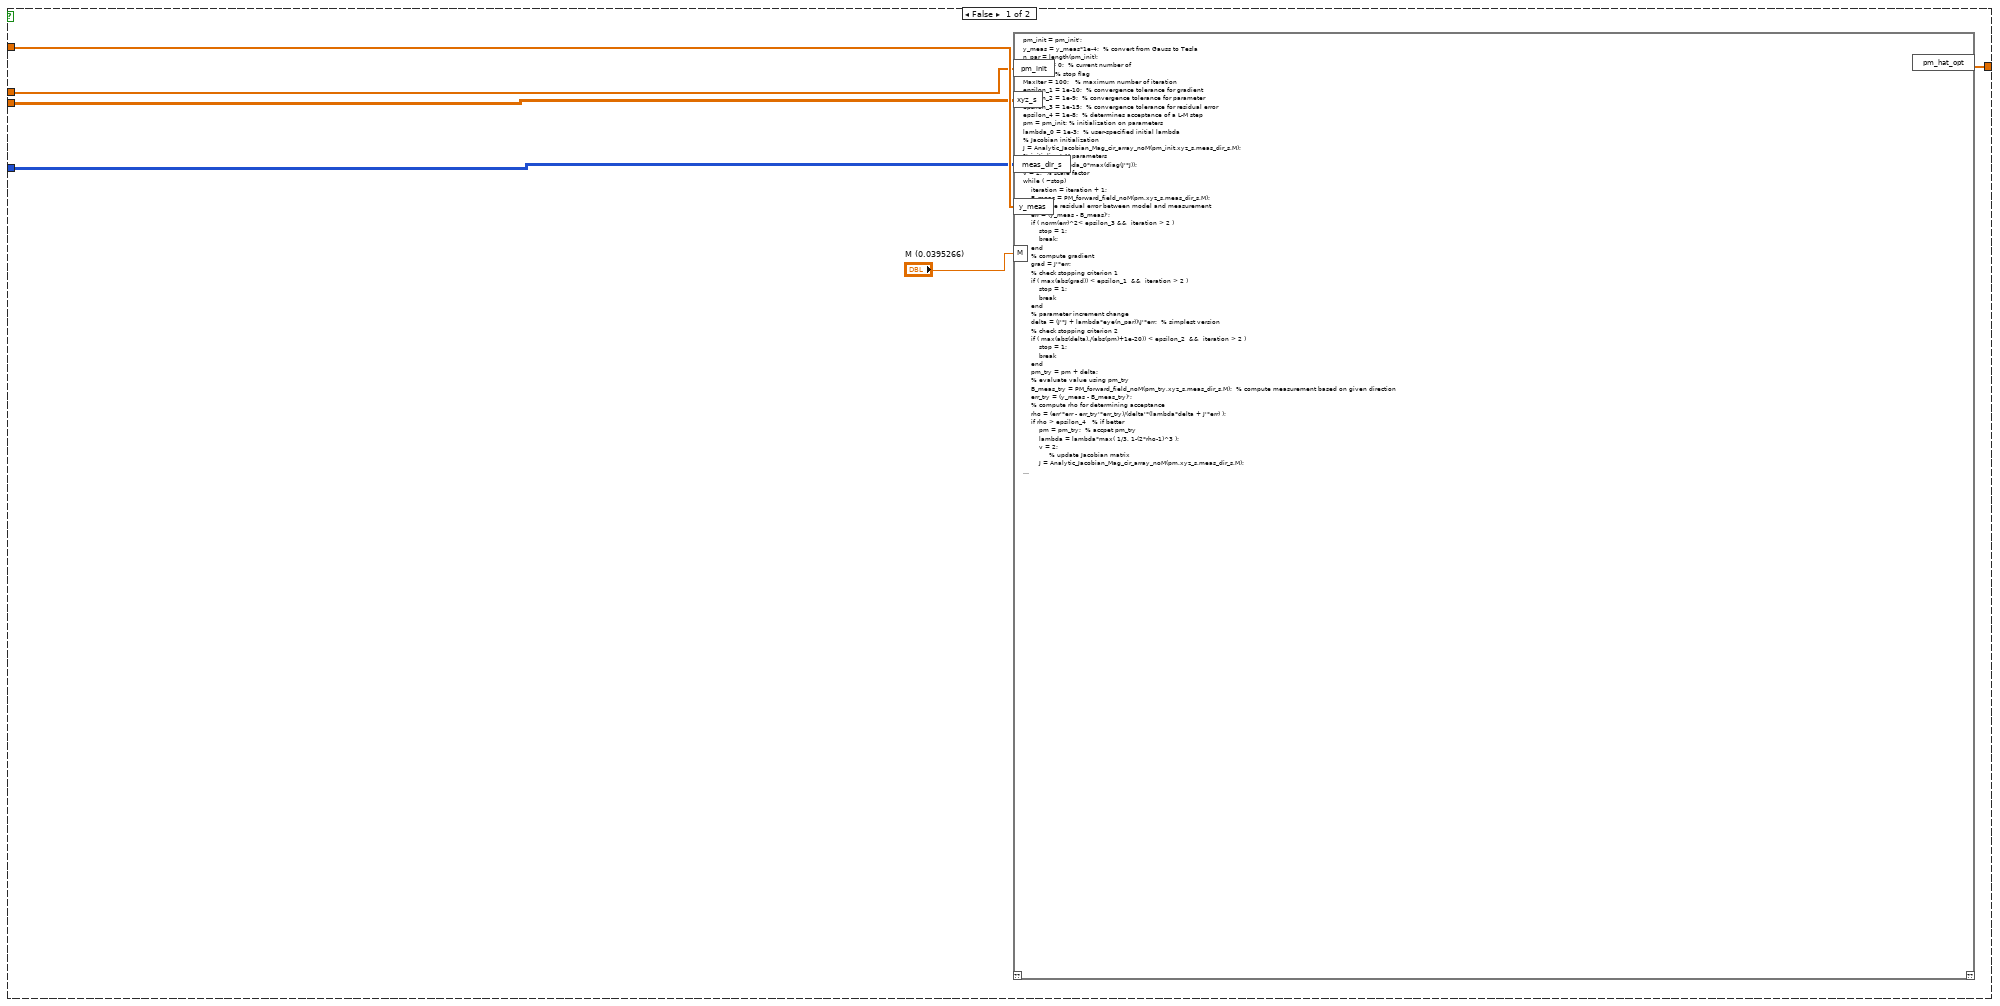
[diagram p7: hidden frame]
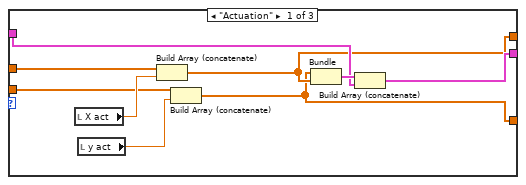
[diagram p8: hidden frame]
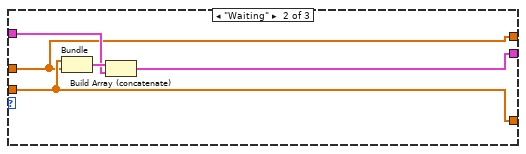
[diagram p9: hidden frame]
diagram:
  # "Intializations"
  # "00 for 2G\n01 for 8G"
  n1 = call <vilib>:"Simple Error Handler.vi"() -> ("error out"=w4:errorcluster)  [unwired: 5 in, 4 out]
  n2 = call <vilib>:"Reset myRIO.vi"("error in (no error)"=w4) -> ()  [unwired: 10 in, 1 out]
  n3 = Reverse 1D Array(array=bool[] [FALSE, TRUE, FALSE, TRUE, TRUE, TRUE, FALSE, TRUE]) -> (reversed array=w17:bool[])
  n4 = Reverse 1D Array(array=bool[] [FALSE, FALSE, FALSE, FALSE, FALSE, FALSE, FALSE, FALSE]) -> (reversed array=w16:bool[])
  n5 = Reverse 1D Array(array=bool[] [FALSE, FALSE, FALSE, FALSE, FALSE, FALSE, FALSE, TRUE]) -> (reversed array=w14:bool[])
  n6 = Boolean Array To Number(Boolean array=w17) -> (number=w11:u32)
  n7 = Boolean Array To Number(Boolean array=w16) -> (number=w10:u32)
  n8 = Boolean Array To Number(Boolean array=w14) -> (number=w9:u32)
  n9 = To Unsigned Byte Integer(number=w11) -> (unsigned 8bit integer=w8:u8)
  n10 = To Unsigned Byte Integer(number=w10) -> (unsigned 8bit integer=w7:u8)
  n11 = To Unsigned Byte Integer(number=w9) -> (unsigned 8bit integer=w6:u8)
  n12 = Build Array(u8 9 ("address"), w8, w7, w6) -> (w5:u8[])
  n13 = flat-sequence {
    tunnel: w5 -> [w40]
    tunnel: [w38] -> w23
    tunnel: [w37] -> w22
    tunnel: [w34] -> w21
    tunnel: [w33] -> w20
    tunnel: [w32] -> w19
    tunnel: [w27] -> w3
    tunnel: [w26] -> w2
    tunnel: [w25] -> w1
    tunnel: w23 -> [w1202]
    tunnel: w22 -> [w1203]
    tunnel: w21 -> [w1204]
    tunnel: w20 -> [w1197]
    tunnel: w19 -> [w1201]
    tunnel: w3 -> [w1200]
    tunnel: w2 -> [w1198]
    tunnel: w1 -> [w1199]
    frame #0 {
      w39 = 8
      # "Initialize the measurement vector to be all 0\nDimension 48x1"
      # "Initializing Sensors"
      n14 = for {
        N: w39 -> [_]
        tunnel: w40 -> [w1028]
        i -> [w1022]
        n15 = Decrement(x=w1022) -> (x-1=w1021:i32)
        n16 = Quotient & Remainder(x=w1021, y=8) -> (x-y*floor(x/y)=w1023:i32)  [unwired: 1 out]
        n17 = Scale By Power Of 2(n=w1023, x=1) -> (x*2^n=w1025:i32)
        n18 = Build Array(w1025) -> (w1031:i32[])
        n19 = xnode "I2C Multiplex 4"("Slave Address (7-bit)"=u8 113, "Bytes to Write"=w1031) -> ("error out"=w1030:errorcluster)  [unwired: 1 in]
        n20 = xnode "I2C Mag Configuration 2"("Slave Address (7-bit)"=u8 13, "Bytes to Write"=w1028, "error in (no error)"=w1030) -> ()  [unwired: 1 out]
      }
      n21 = for {
        N: w39 -> [_]
        tunnel: w40 -> [w1115]
        i -> [w1109]
        n22 = Decrement(x=w1109) -> (x-1=w1108:i32)
        n23 = Quotient & Remainder(x=w1108, y=8) -> (x-y*floor(x/y)=w1110:i32)  [unwired: 1 out]
        n24 = Scale By Power Of 2(n=w1110, x=1) -> (x*2^n=w1112:i32)
        n25 = Build Array(w1112) -> (w1118:i32[])
        n26 = xnode "I2C Multiplex"("Slave Address (7-bit)"=u8 112, "Bytes to Write"=w1118) -> ("error out"=w1117:errorcluster)  [unwired: 1 in]
        n27 = xnode "I2C Mag Configuration"("Slave Address (7-bit)"=u8 13, "Bytes to Write"=w1115, "error in (no error)"=w1117) -> ()  [unwired: 1 out]
      }
      n28 = mathscript code="magnet_distance = 54;\n\n%xyz_s = [0.0612777298600452 0.0612777298600452 0.0612777298600452 0.0613339046214879 0.0613339046214879 0.0613339046214879 0.0617519169616129 0.0617519169616129 0.0617519169616129 0.0617278031895696 0.0617278031895696 0.0617278031895696 -0.00167587448144978 -0.00167587448144978 -0.00167587448144978 0.000602084909327022 0.000602084909327022 0.000602084909327022 0.00188819008475229 0.00188819008475229 0.00188819008475229 0.00165227304665085 0.00165227304665085 0.00165227304665085 -0.0606370242471406 -0.0606370242471406 -0.0606370242471406 -0.0611347541127161 -0.0611347541127161 -0.0611347541127161 -0.0611396275851359 -0.0611396275851359 -0.0611396275851359 -0.0607066251575206 -0.0607066251575206 -0.0607066251575206 -0.00174297673440637 -0.00174297673440637 -0.00174297673440637 -0.000184533688514991 -0.000184533688514991 -0.000184533688514991 0.00203926333921812 0.00203926333921812 0.00203926333921812 0.00389433540899126 0.00389433540899126 0.00389433540899126;-0.0383039026828955 -0.0383039026828955 -0.0383039026828955 -0.012806715187076 -0.012806715187076 -0.012806715187076 0.0122506598898495 0.0122506598898495 0.0122506598898495 0.0373597708961822 0.0373597708961822 0.0373597708961822 -0.0395839775993431 -0.0395839775993431 -0.0395839775993431 -0.0142163399313766 -0.0142163399313766 -0.0142163399313766 0.0107770086004868 0.0107770086004868 0.0107770086004868 0.0365600556411557 0.0365600556411557 0.0365600556411557 -0.040094901607281 -0.040094901607281 -0.040094901607281 -0.0149090266343068 -0.0149090266343068 -0.0149090266343068 0.0107078118967093 0.0107078118967093 0.0107078118967093 0.0356978973873521 0.0356978973873521 0.0356978973873521 -0.0392056799428433 -0.0392056799428433 -0.0392056799428433 -0.0139322320487061 -0.0139322320487061 -0.0139322320487061 0.0112429513248133 0.0112429513248133 0.0112429513248133 0.0361205812401305 0.0361205812401305 0.0361205812401305;0.00307213814961651 0.00307213814961651 0.00307213814961651 0.0033242461093476 0.0033242461093476 0.0033242461093476 0.00389293419390068 0.00389293419390068 0.00389293419390068 0.00390199978115286 0.00390199978115286 0.00390199978115286 0.0640688323293379 0.0640688323293379 0.0640688323293379 0.0636929900573754 0.0636929900573754 0.0636929900573754 0.0635181326061399 0.0635181326061399 0.0635181326061399 0.0633759954094267 0.0633759954094267 0.0633759954094267 -0.00381527257187291 -0.00381527257187291 -0.00381527257187291 -0.00312975643341264 -0.00312975643341264 -0.00312975643341264 -0.00272771938684928 -0.00272771938684928 -0.00272771938684928 -0.00268843620404175 -0.00268843620404175 -0.00268843620404175 -0.0628805002941716 -0.0628805002941716 -0.0628805002941716 -0.063138590462401 -0.063138590462401 -0.063138590462401 -0.063695098330538 -0.063695098330538 -0.063695098330538 -0.0638823957044235 -0.0638823957044235 -0.0638823957044235]\n\nxyz_s = [0.0548336907197902\t0.0548336907197902\t0.0548336907197902\t0.0546405013356616\t0.0546405013356616\t0.0546405013356616\t0.0550964103281113\t0.0550964103281113\t0.0550964103281113\t0.0549474800958512\t0.0549474800958512\t0.0549474800958512\t-0.00131873321916003\t-0.00131873321916003\t-0.00131873321916003\t-0.000391192401749352\t-0.000391192401749352\t-0.000391192401749352\t-0.000486879515597376\t-0.000486879515597376\t-0.000486879515597376\t-0.000608055705082732\t-0.000608055705082732\t-0.000608055705082732\t-0.0541791813007843\t-0.0541791813007843\t-0.0541791813007843\t-0.0539989087386222\t-0.0539989087386222\t-0.0539989087386222\t-0.0544048450277662\t-0.0544048450277662\t-0.0544048450277662\t-0.0542370658799858\t-0.0542370658799858\t-0.0542370658799858\t0.000325153844385146\t0.000325153844385146\t0.000325153844385146\t0.00287727553963575\t0.00287727553963575\t0.00287727553963575\t0.00440239104583381\t0.00440239104583381\t0.00440239104583381\t0.00434430183335338\t0.00434430183335338\t0.00434430183335338\n-0.0384825013167492\t-0.0384825013167492\t-0.0384825013167492\t-0.0133656742318122\t-0.0133656742318122\t-0.0133656742318122\t0.0107590038833561\t0.0107590038833561\t0.0107590038833561\t0.0363501381761792\t0.0363501381761792\t0.0363501381761792\t-0.0407206389319919\t-0.0407206389319919\t-0.0407206389319919\t-0.0153413650284744\t-0.0153413650284744\t-0.0153413650284744\t0.00915776152329285\t0.00915776152329285\t0.00915776152329285\t0.0348169163075068\t0.0348169163075068\t0.0348169163075068\t-0.0399169117606167\t-0.0399169117606167\t-0.0399169117606167\t-0.0148677892825094\t-0.0148677892825094\t-0.0148677892825094\t0.0103245638209904\t0.0103245638209904\t0.0103245638209904\t0.0358526178908690\t0.0358526178908690\t0.0358526178908690\t-0.0386092596443539\t-0.0386092596443539\t-0.0386092596443539\t-0.0137960900850645\t-0.0137960900850645\t-0.0137960900850645\t0.0116482464104805\t0.0116482464104805\t0.0116482464104805\t0.0361285130175356\t0.0361285130175356\t0.0361285130175356\n-0.000550076753147838\t-0.000550076753147838\t-0.000550076753147838\t0.000739706630282587\t0.000739706630282587\t0.000739706630282587\t0.00200581187624003\t0.00200581187624003\t0.00200581187624003\t0.00195674567089956\t0.00195674567089956\t0.00195674567089956\t0.0523038155150723\t0.0523038155150723\t0.0523038155150723\t0.0522221453682739\t0.0522221453682739\t0.0522221453682739\t0.0522386769210956\t0.0522386769210956\t0.0522386769210956\t0.0519828704003945\t0.0519828704003945\t0.0519828704003945\t-0.00507159747123124\t-0.00507159747123124\t-0.00507159747123124\t-0.00263114160414311\t-0.00263114160414311\t-0.00263114160414311\t-0.00206958862952268\t-0.00206958862952268\t-0.00206958862952268\t-0.00198663238644750\t-0.00198663238644750\t-0.00198663238644750\t-0.0573644024378140\t-0.0573644024378140\t-0.0573644024378140\t-0.0567248385214366\t-0.0567248385214366\t-0.0567248385214366\t-0.0563512780514148\t-0.0563512780514148\t-0.0563512780514148\t-0.0561807916479818\t-0.0561807916479818\t-0.0561807916479818];\n\nmeas_dir_s = [mirrorh(diag([1;-1;1])),...\n              mirrorh(diag([1;-1;1])),...\n              mirrorh(diag([1;-1;1])),...\n              mirrorh(diag([1;-1;1])),...\n              diag([-1;-1;1]),...\n              diag([-1;-1;1]),...\n              diag([-1;-1;1]),...\n              diag([-1;-1;1]),...\n              mirrorh(diag([-1;-1;-1])),...\n              mirrorh(diag([-1;-1;-1])),...\n              mirrorh(diag([-1;-1;-1])),...\n              mirrorh(diag([-1;-1;-1])),... \n              diag([1;-1;-1]),...\n              diag([1;-1;-1]),...\n              diag([1;-1;-1]),...\n              diag([1;-1;-1])];\n\npm_init = [0;0;0;pi/2;-pi/2;0.04];\n\nB_earth = [-0.387793651\t-0.429301587\t-0.024730159...\n-0.463698413\t-0.463777778\t-0.006666667...\n-0.475349206\t-0.45947619\t-0.025063492...\n-0.401539683\t-0.412460317\t-0.074888889...\n0.059603175\t-0.338349206\t-0.332396825...\n-0.068809524\t-0.464920635\t-0.238555556...\n0.024650794\t-0.417619048\t-0.312857143...\n0.005253968\t-0.392142857\t-0.383603175...\n0.275380952\t-0.378952381\t0.058444444...\n0.174258065\t-0.407048387\t0.188903226...\n0.215741935\t-0.484370968\t0.149596774...\n0.320645161\t-0.386774194\t0.065709677...\n-0.087888889\t-0.282650794\t0.306793651...\n-0.114096774\t-0.323032258\t0.365322581...\n-0.060806452\t-0.210467742\t0.355...\n-0.128741935\t-0.226709677\t0.308935484];"() -> ("meas_dir_s"=w38:i32[][], "xyz_s"=w37:dbl[][], "pm_init"=w33:dbl[], "B_earth"=w32:dbl[])  [unwired: 1 in, 1 out]
      n29 = case shown="\"Branch off\"" "Enum" {
        tunnel: [w41 w180 w477] -> w27
        frame "Curved Path" {
          n30 = mathscript code="% line 1\ny1=[-35:0.1:0];\nx1=sqrt(35.92^2-(y1+17.5).^2)-26.37-1;\n\ny2=[-35:0.1:0];\nx2 =sqrt(35.92^2-(y1+17.5).^2)-26.37-10+1;\n\ny3 = [0:0.1:35];\nx3 = -sqrt(35.92^2-(y3-17.5).^2)+36.37-1;\n\ny4 = [0:0.1:35];\nx4 = -sqrt(35.92^2-(y4-17.5).^2)+36.37-10+1;"() -> ("y1"=w53:dbl[], "x1"=w52:cdb[], "y2"=w50:dbl[], "x2"=w49:cdb[], "y3"=w48:dbl[], "x3"=w47:cdb[], "y4"=w46:dbl[], "x4"=w45:cdb[])  [unwired: 1 in, 1 out]
          n31 = Bundle("y1"=w53, "x1"=w52) -> (w51:cluster{"y1":dbl[], "x1":cdb[]})  [unwired: 1 in]
          n32 = Bundle("y2"=w50, "x2"=w49) -> (w44:cluster{"y2":dbl[], "x2":cdb[]})  [unwired: 1 in]
          n33 = Bundle("y3"=w48, "x3"=w47) -> (w43:cluster{"y3":dbl[], "x3":cdb[]})  [unwired: 1 in]
          n34 = Bundle("y4"=w46, "x4"=w45) -> (w42:cluster{"y4":dbl[], "x4":cdb[]})  [unwired: 1 in]
          n35 = Build Array(w51, w44, w43, w42) -> (w41:cluster{"y4":dbl[], "x4":cdb[]}[])
        }
        frame "Bifurcation" {
          # "For plotting"
          n36 = mathscript code="width = 6;\nlen = 80;\ny_offset= sqrt(width^2 - (width/2)^2)\nx_offset = width/2\n\n\n% line 1\nhorizontal_y = [y_offset:0.1:len];\ny1 = horizontal_y;\nx1 = -x_offset*ones(1,length(y1));\n\n% line 2\ny2 =horizontal_y;\nx2 = x_offset*ones(1,length(y1));\n\n%line 3\ny_center_slope = [-len:0.1:y_offset];\nx_center_slope = -(1/3)*(y_center_slope-y_offset) + x_offset;\n\nx11 = x_center_slope;\ny11 = y_center_slope;\n\nx22 = -x_center_slope;\ny22 = y_center_slope;\n\n% line 3\ny_side_slope = [-len:0.1:0];\nx_center_slope = -(1/3)*y_side_slope;\n\nx3 = -x_center_slope;\ny3 = y_side_slope;\n\n% line 4\nx4 = x_center_slope;\ny4 = y_side_slope;"() -> ("y1"=w198:dbl[], "x1"=w197:dbl[], "y11"=w196:dbl[], "x11"=w195:cdb[], "y2"=w192:dbl[], "x2"=w191:dbl[], "y22"=w189:dbl[], "x22"=w188:cdb[], "y3"=w186:dbl[], "x3"=w185:dbl[], "y4"=w183:dbl[], "x4"=w182:dbl[])  [unwired: 1 in, 1 out]
          n37 = Bundle("y1"=w198, "x1"=w197) -> (w194:cluster{"y1":dbl[], "x1":dbl[]})  [unwired: 1 in]
          n38 = Bundle("y11"=w196, "x11"=w195) -> (w193:cluster{"y11":dbl[], "x11":cdb[]})  [unwired: 1 in]
          n39 = Bundle("y2"=w192, "x2"=w191) -> (w190:cluster{"y2":dbl[], "x2":dbl[]})  [unwired: 1 in]
          n40 = Bundle("y22"=w189, "x22"=w188) -> (w187:cluster{"y22":dbl[], "x22":cdb[]})  [unwired: 1 in]
          n41 = Bundle("y3"=w186, "x3"=w185) -> (w184:cluster{"y3":dbl[], "x3":dbl[]})  [unwired: 1 in]
          n42 = Bundle("y4"=w183, "x4"=w182) -> (w181:cluster{"y4":dbl[], "x4":dbl[]})  [unwired: 1 in]
          n43 = Build Array(w194, w193, w190, w187, w184, w181) -> (w180:cluster{"y4":dbl[], "x22":cdb[]}[])
        }
        frame "Branch off" {
          # "For plotting"
          n44 = mathscript code="width = 6;\nlen = 80;\ny_offset= width/sin(0.5236)\nx_offset = width/2\nbranch = 20\n\n\n% line 1 straight pos\nhorizontal_y = [y_offset+branch:0.1:len];\ny1 = horizontal_y;\nx1 = x_offset*ones(1,length(y1));\n\n% line 2 straight long\ny2 =[-len:0.1:len];\nx2 = -x_offset*ones(1,length(y2));\n\n%line 3\ny_center_slope = [-len:0.1:0+branch];\nx_center_slope = -(1/3)*(y_center_slope-branch) + x_offset;\n\ny11 = y_center_slope;\nx11 = x_center_slope;\n\n\ny_side_slope = [-len:0.1:y_offset+branch];\nx_side_slope = -(1/3)*(y_side_slope - y_offset-branch) + x_offset ;\nx22 = x_side_slope;\ny22 = y_side_slope;\n\n% line 3\ny3 = [-len:0.1:0+branch];\nx3 = x_offset*ones(1,length(y3));\n\n\n% line 4\nx4 = x1;\ny4 = y1;"() -> ("y1"=w495:dbl[], "x1"=w494:dbl[], "y11"=w493:dbl[], "x11"=w492:dbl[], "y2"=w489:dbl[], "x2"=w488:dbl[], "y22"=w486:dbl[], "x22"=w485:dbl[], "y3"=w483:dbl[], "x3"=w482:dbl[], "y4"=w480:dbl[], "x4"=w479:dbl[])  [unwired: 1 in, 1 out]
          n45 = Bundle("y1"=w495, "x1"=w494) -> (w491:cluster{"y1":dbl[], "x1":dbl[]})  [unwired: 1 in]
          n46 = Bundle("y11"=w493, "x11"=w492) -> (w490:cluster{"y11":dbl[], "x11":dbl[]})  [unwired: 1 in]
          n47 = Bundle("y2"=w489, "x2"=w488) -> (w487:cluster{"y2":dbl[], "x2":dbl[]})  [unwired: 1 in]
          n48 = Bundle("y22"=w486, "x22"=w485) -> (w484:cluster{"y22":dbl[], "x22":dbl[]})  [unwired: 1 in]
          n49 = Bundle("y3"=w483, "x3"=w482) -> (w481:cluster{"y3":dbl[], "x3":dbl[]})  [unwired: 1 in]
          n50 = Bundle("y4"=w480, "x4"=w479) -> (w478:cluster{"y4":dbl[], "x4":dbl[]})  [unwired: 1 in]
          n51 = Build Array(w491, w490, w487, w484, w481, w478) -> (w477:cluster{"y4":dbl[], "x4":dbl[]}[])
        }
      }
      n52 = Initialize Array(0.0 ("element"), 0 ("dimension size")) -> (w26:dbl[])
      n53 = Initialize Array(0.0 ("element"), 0 ("dimension size")) -> (w25:dbl[])
      n54 = Initialize Array(0.0 ("element"), 48 ("dimension size")) -> (w34:dbl[])
    }
    frame #1 {
      # "Plotting"
      n55 = while {
        shift-right: [w3718] -> _
        shift-left: w1198 -> [w3713]
        shift-right: [w3719] -> _
        shift-left: w1199 -> [w3710]
        tunnel: w1200 -> [w3715]
        tunnel: w1198 -> [w3708]
        stop <- w3714 stop-if-true
        n56 = call "Wait"("Count(mSec)"=u32 250) -> ()  [unwired: 1 out]
        n57 = local read "Action Mode"() -> (w3716:T2)
        n58 = Select(t=w3708, s="Clear plot?", f=w3713) -> (s? t:f=w3712:dbl[])
        n59 = Select(t=w3708, s="Clear plot?", f=w3710) -> (s? t:f=w3709:dbl[])
        n60 = case shown="\"Sensing\", Default" w3716 {
          tunnel: w3712 -> [w3726 w3730 w3748]
          tunnel: w3709 -> [w3723 w3731 w3747]
          tunnel: [w3721 w3731 w3746] -> w3719
          tunnel: [w3724 w3730 w3745] -> w3718
          tunnel: [w3728 w3733 w3740] -> w3717
          tunnel: w3715 -> [w3727 w3732 w3735]
          frame "Actuation" {
            n61 = local read "X act"() -> (w3725:dbl)
            n62 = local read "y act"() -> (w3722:dbl)
            n63 = Build Array (concatenate)(w3726, w3725) -> (w3724:dbl[])
            n64 = Build Array (concatenate)(w3723, w3722) -> (w3721:dbl[])
            n65 = Bundle(w3721, w3724) -> (w3729:cluster{dbl[], dbl[]})  [unwired: 1 in]
            n66 = Build Array (concatenate)(w3729, w3727) -> (w3728:cluster{"y4":dbl[], "x22":cdb[]}[])
          }
          frame "Waiting" {
            n67 = Bundle(w3731, w3730) -> (w3734:cluster{dbl[], dbl[]})  [unwired: 1 in]
            n68 = Build Array (concatenate)(w3734, w3732) -> (w3733:cluster{"y4":dbl[], "x22":cdb[]}[])
          }
          frame "Sensing", Default {
            # "X"
            # "Y"
            n69 = local read "pm_hat_opt"() -> (w3738:dbl[])
            n70 = Index Array(array=w3738, index #1=0 ("index"), index #2=1 ("index")) -> (element #1=w3737:dbl, element #2=w3736:dbl)
            n71 = Multiply(x=1000.0, y=w3737) -> (x*y=w3741:dbl)
            n72 = Multiply(x=w3736, y=-1000.0) -> (x*y=w3743:dbl)
            n73 = Build Array (concatenate)(w3748, w3741) -> (w3745:dbl[])
            n74 = Build Array (concatenate)(w3747, w3743) -> (w3746:dbl[])
            n75 = Bundle(w3746, w3745) -> (w3739:cluster{dbl[], dbl[]})  [unwired: 1 in]
            n76 = Build Array (concatenate)(w3739, w3735) -> (w3740:cluster{"y4":dbl[], "x22":cdb[]}[])
          }
        }
        "XY Graph" <- w3717
        n77 = local read "stop"() -> (w3714:bool)
      }
      n78 = local read "Update M in realtime?"() -> (w1195:bool)
      n79 = case shown="True" w1195 {
        tunnel: [w1205 w1217] -> w1196
        tunnel: w1197 -> [w1216 w1217]
        frame False {
          n80 = Index Array(array=w1216, index #1=0 ("index"), index #2=1 ("index"), index #3=2 ("index"), index #4=3 ("index"), index #5=4 ("index")) -> (element #1=w1210:dbl, element #2=w1209:dbl, element #3=w1208:dbl, element #4=w1207:dbl, element #5=w1206:dbl)
          n81 = Build Array(w1210, w1209, w1208, w1207, w1206) -> (w1205:dbl[])
        }
        frame True {
        }
      }
      n82 = while {
        shift-right: [w1220] -> _
        shift-left: w1204 -> [w1226]
        shift-right: [w1225] -> _
        shift-left: w1196 -> [w1224]
        tunnel: w1203 -> [w1223]
        tunnel: w1202 -> [w1222]
        tunnel: w1201 -> [w1221]
        stop <- "stop" stop-if-true
        n83 = case shown="\"Actuation\"" "Action Mode" {
          tunnel: w1226 -> [w1301 w1492 w1543]
          tunnel: [w1299 w1493 w1542] -> w1225
          tunnel: w1224 -> [w1300 w1493 w1541]
          tunnel: w1223 -> [_ _ w1540]
          tunnel: w1222 -> [_ _ w1539]
          tunnel: w1221 -> [_ _ w1538]
          tunnel: [w1301 w1492 w1537] -> w1220
          frame "Actuation" {
            n84 = flat-sequence {
              tunnel: w1300 -> [w1335]
              tunnel: [w1335] -> w1299
              frame #0 {
                w1317 = 22.0  # length
                n85 = xnode "Analog input (1 sample) 3"() -> ("C/AI0 (AI0)"=w1309:dbl)  [unwired: 1 in, 1 out]
                "Feed Encoder 2" <- w1309
                n86 = xnode "Analog input (1 sample) 3"() -> ("SteeringInput (C/AI1 (AI1))"=w1340:dbl)  [unwired: 1 in, 1 out]
                "Steer Encoder" <- w1340
                n87 = call "Wait2"("Count(uSec)"=u32 1000 ("Count(mSec)")) -> ()  [unwired: 1 out]
                n88 = Divide(x=w1309, y=0.004883) -> (x/y=w1310:dbl)
                n89 = Multiply(x=w1310, y=-0.0172) -> (x*y=w1311:dbl)
                n90 = Divide(x=w1340, y=10.0) -> (x/y=w1339:dbl)
                "Duty Ratio" <- w1339
                n91 = Select(t=w1339, s="Actuation on?", f=0.0) -> (s? t:f=w1344:dbl)
                n92 = Absolute Value(x=w1344) -> (abs(x)=w1345:dbl)
                n93 = Multiply(x=w1311, y="Steer Gain (2.3)") -> (x*y=w1306:dbl)
                "feed displacement" <- w1306
                n94 = xnode "PWM 2"("Duty Cycle"=w1345) -> ()  [unwired: 1 in, 1 out]
                n95 = Greater Than 0?(x=w1344) -> (x > 0?=w1343:bool)
                n96 = xnode "Digital output (1 sample)"("C/DIO2 (DIO2)"=w1343) -> ()  [unwired: 1 in, 1 out]
                n97 = Multiply(x=w1339, y=43.04367) -> (x*y=w1337:dbl)
                n98 = Add(x=w1337, y=0.48195) -> (x+y=w1330:dbl)
                "Degree Angle" <- w1330
                n99 = Multiply(x=3.141592653589793, y=w1330) -> (x*y=w1328:dbl)
                n100 = Divide(x=w1328, y=180.0) -> (x/y=w1323:dbl)
                n101 = Sine(x=w1323) -> (sin(x)=w1322:dbl)
                n102 = Cosine(x=w1323) -> (cos(x)=w1325:dbl)
                n103 = Index Array(array=w1335, index #1=0 ("index"), index #2=1 ("index")) -> (element #1=w1332:dbl, element #2=w1331:dbl)
                n104 = Multiply(x=w1322, y=w1317) -> (x*y=w1321:dbl)
                "delta x" <- w1321
                n105 = Multiply(x=w1325, y=w1317) -> (x*y=w1315:dbl)
                n106 = Multiply(x=-1.0, y=w1317) -> (x*y=w1313:dbl)
                n107 = Subtract(x=w1306, y=w1313) -> (x-y=w1326:dbl)
                n108 = Multiply(x=w1331, y=0.0) -> (x*y=w1304:dbl)
                n109 = Multiply(x=-1.0, y=w1315) -> (x*y=w1314:dbl)
                n110 = Add(x=w1314, y=w1326) -> (x+y=w1324:dbl)
                "delta Y" <- w1324
                n111 = Multiply(x=1000.0, y=w1332) -> (x*y=w1305:dbl)
                n112 = Add(x=w1305, y=w1321) -> (x+y=→"X act":dbl)
                n113 = Add(x=w1304, y=w1324) -> (x+y=→"y act":dbl)
              }
            }
          }
          frame "Waiting" {
            # "Change to next Sensing mode"
            # "Gradually decrease to zero"
            # "wait for field to disappear"
            n114 = flat-sequence {
              frame #0 {
                n115 = local write "Actuation on?"(FALSE ("Actuation on?")) -> ()
                n116 = call "Wait3"("Count(mSec)"=u32 60) -> ()  [unwired: 1 out]
                n117 = local write "Reset Actuation"(TRUE ("Reset Actuation")) -> ()
                n118 = xnode "PWM"("Duty Cycle"=0.0) -> ()  [unwired: 1 in, 1 out]
              }
              frame #1 {
                n119 = local write "Reset Actuation"(FALSE ("Reset Actuation")) -> ()
              }
            }
          }
          frame "Sensing", Default {
            n120 = call "Tick Count"() -> ("Tick Count(uSec)"=w1536:u32)
            n121 = feedback #1() -> (w1535:u32)  [unwired: 1 in]
            n122 = feedback-in #1(w1536) -> ()
            n123 = flat-sequence {
              tunnel: [w1546] -> w1544
              tunnel: w1543 -> [w1545]
              tunnel: w1544 -> [w1786]
              tunnel: [w1790] -> w1542
              tunnel: w1541 -> [w1789]
              tunnel: w1540 -> [w1788]
              tunnel: w1539 -> [w1787]
              tunnel: w1538 -> [w1784]
              tunnel: [w1786] -> w1537
              frame #0 {
                # "Run 8 Iterations to read all sensors data simultaneously"
                n124 = for {
                  N: 8 -> [_]
                  shift-right: [w1559] -> w1546
                  shift-left: w1545 -> [w1561]
                  i -> [w1562]
                  # "B_meas"
                  n125 = Decrement(x=w1562) -> (x-1=w1555:i32)
                  n126 = Quotient & Remainder(x=w1555, y=8) -> (x-y*floor(x/y)=w1563:i32)  [unwired: 1 out]
                  n127 = Less Or Equal?(x=w1555, y=3) -> (x <= y?=w1553:bool)
                  n128 = Multiply(x=w1555, y=3) -> (x*y=w1552:i32)
                  n129 = Scale By Power Of 2(n=w1563, x=1) -> (x*2^n=w1564:i32)
                  n130 = Select(t=0, s=w1553, f=24) -> (s? t:f=w1549:i32)
                  n131 = Add(x=w1552, y=12) -> (x+y=w1556:i32)
                  n132 = Add(x=w1552, y=w1549) -> (x+y=w1548:i32)
                  n133 = Build Array(w1564) -> (w1566:i32[])
                  n134 = flat-sequence {
                    tunnel: w1566 -> [w1579]
                    tunnel: [w1579] -> w1569
                    tunnel: [w1577] -> w1568
                    tunnel: w1561 -> [w1573]
                    tunnel: [w1572] -> w1560
                    tunnel: w1556 -> [w1570]
                    tunnel: w1569 -> [w1686]
                    tunnel: w1568 -> [w1684]
                    tunnel: w1560 -> [w1683]
                    tunnel: [w1682] -> w1559
                    tunnel: w1548 -> [w1677]
                    frame #0 {
                      w1588 = i16 3000  # Gain Lsb/G
                      # "Sensor 5,6,7,8,9,10,11,12"
                      # "Z"
                      # "Y"
                      # "X"
                      n135 = xnode "I2C Multiplex 2"("Slave Address (7-bit)"=u8 112, "Bytes to Write"=w1579) -> ("error out"=w1578:errorcluster)  [unwired: 1 in]
                      n136 = Build Array(u8 0) -> (w1592:u8[])
                      n137 = xnode "I2C 2"("Slave Address (7-bit)"=u8 13, "Bytes to Write"=w1592, "Byte Count"=u32 6, "error in (no error)"=w1578) -> ("Bytes Read"=w1595:u8[], "error out"=w1577:errorcluster)
                      n138 = Index Array(array=w1595) -> (element #1=w1587:u8, element #2=w1586:u8, element #3=w1584:u8, element #4=w1585:u8, element #5=w1582:u8, element #6=w1583:u8)  [unwired: 6 in]
                      n139 = Join Numbers(hi=w1586, lo=w1587) -> ((hi.lo)=w1598:u16)
                      n140 = Join Numbers(hi=w1585, lo=w1584) -> ((hi.lo)=w1596:u16)
                      n141 = Join Numbers(hi=w1583, lo=w1582) -> ((hi.lo)=w1597:u16)
                      n142 = To Word Integer(number=w1598) -> (16bit integer=w1591:i16)
                      n143 = To Word Integer(number=w1596) -> (16bit integer=w1590:i16)
                      n144 = To Word Integer(number=w1597) -> (16bit integer=w1589:i16)
                      n145 = Divide(x=w1591, y=w1588) -> (x/y=w1576:dbl)
                      n146 = Divide(x=w1590, y=w1588) -> (x/y=w1575:dbl)
                      n147 = Divide(x=w1589, y=w1588) -> (x/y=w1574:dbl)
                      n148 = Build Array(w1576, w1575, w1574) -> (w1571:dbl[])
                      n149 = Replace Array Subset(array=w1573, new element=w1571, index=w1570) -> (w1572:dbl[])
                    }
                    frame #1 {
                      w1695 = i16 3000  # Gain Lsb/G
                      # "Sensor 1,2,3,4,13,14,15,16"
                      n150 = xnode "I2C Multiplex 3"("Slave Address (7-bit)"=u8 113, "Bytes to Write"=w1686, "error in (no error)"=w1684) -> ("error out"=w1685:errorcluster)
                      n151 = Build Array(u8 0) -> (w1699:u8[])
                      n152 = xnode "I2C"("Slave Address (7-bit)"=u8 13, "Bytes to Write"=w1699, "Byte Count"=u32 6, "error in (no error)"=w1685) -> ("Bytes Read"=w1702:u8[])  [unwired: 1 out]
                      n153 = Index Array(array=w1702) -> (element #1=w1694:u8, element #2=w1693:u8, element #3=w1691:u8, element #4=w1692:u8, element #5=w1689:u8, element #6=w1690:u8)  [unwired: 6 in]
                      n154 = Join Numbers(hi=w1693, lo=w1694) -> ((hi.lo)=w1705:u16)
                      n155 = Join Numbers(hi=w1692, lo=w1691) -> ((hi.lo)=w1703:u16)
                      n156 = Join Numbers(hi=w1690, lo=w1689) -> ((hi.lo)=w1704:u16)
                      n157 = To Word Integer(number=w1705) -> (16bit integer=w1698:i16)
                      n158 = To Word Integer(number=w1703) -> (16bit integer=w1697:i16)
                      n159 = To Word Integer(number=w1704) -> (16bit integer=w1696:i16)
                      n160 = Divide(x=w1698, y=w1695) -> (x/y=w1681:dbl)
                      n161 = Divide(x=w1697, y=w1695) -> (x/y=w1680:dbl)
                      n162 = Divide(x=w1696, y=w1695) -> (x/y=w1679:dbl)
                      n163 = Build Array(w1681, w1680, w1679) -> (w1678:dbl[])
                      n164 = Replace Array Subset(array=w1683, new element=w1678, index=w1677) -> (w1682:dbl[])
                    }
                  }
                }
              }
              frame #1 {
                # "B_earth_field"
                n165 = Subtract(x=w1786, y=w1784) -> (x-y=w1791:dbl[])
                n166 = case shown="True" "Update M in realtime?" {
                  tunnel: w1791 -> [w1796 w2761]
                  tunnel: [w1792 w2760] -> w1790
                  tunnel: w1789 -> [w1793 w2759]
                  tunnel: w1788 -> [w1794 w2758]
                  tunnel: w1787 -> [w1795 w2757]
                  frame False {
                    n167 = mathscript code="pm_init = pm_init';\ny_meas = y_meas*1e-4;  % convert from Gauss to Tesla\nn_par = length(pm_init);\niteration = 0;  % current number of \nstop = 0;  % stop flag\nMaxIter = 100;   % maximum number of iteration\nepsilon_1 = 1e-10;  % convergence tolerance for gradient\nepsilon_2 = 1e-9;  % convergence tolerance for parameter\nepsilon_3 = 1e-15;  % convergence tolerance for residual error\nepsilon_4 = 1e-8;  % determines acceptance of a L-M step\npm = pm_init; % initialization on parameters\nlambda_0 = 1e-3;  % user-specified initial lambda\n% Jacobian initialization\nJ = Analytic_Jacobian_Mag_cir_array_noM(pm_init,xyz_s,meas_dir_s,M);\n% initialize L-M parameters\nlambda = lambda_0*max(diag(J'*J));\nv = 2;  % scale factor\nwhile ( ~stop)\n    iteration = iteration + 1;\n    B_meas = PM_forward_field_noM(pm,xyz_s,meas_dir_s,M);\n% compute residual error between model and measurement\n    err = (y_meas - B_meas)';\n    if ( norm(err)^2< epsilon_3 &&  iteration > 2 )\n        stop = 1;\n        break;\n    end\n    % compute gradient\n    grad = J'*err;\n    % check stopping criterion 1\n    if ( max(abs(grad)) < epsilon_1  &&  iteration > 2 )\n        stop = 1;\n        break\n    end\n    % parameter increment change\n    delta = (J'*J + lambda*eye(n_par))\\J'*err;  % simplest version\n    % check stopping criterion 2 \n    if ( max(abs(delta)./(abs(pm)+1e-20)) < epsilon_2  &&  iteration > 2 )\n        stop = 1;\n        break\n    end\n    pm_try = pm + delta;\n    % evaluate value using pm_try\n    B_meas_try = PM_forward_field_noM(pm_try,xyz_s,meas_dir_s,M);  % compute measurement based on given direction\n    err_try = (y_meas - B_meas_try)';\n    % compute rho for determining acceptance\n    rho = (err'*err - err_try'*err_try)/(delta'*(lambda*delta + J'*err) );\n    if rho > epsilon_4   % if better\n        pm = pm_try;  % accpet pm_try\n        lambda = lambda*max( 1/3, 1-(2*rho-1)^3 );\n        v = 2;\n             % update Jacobian matrix\n        J = Analytic_Jacobian_Mag_cir_array_noM(pm,xyz_s,meas_dir_s,M);\n    else      % if not better\n        lambda = lambda*v;\n        v = 2*v;\n    end\n    if ( iteration == MaxIter )\n        stop = 1;\n    end\nend\n\npm_hat_opt = pm;"("meas_dir_s"=w1795, "xyz_s"=w1794, "y_meas"=w1796, "pm_init"=w1793, "M"="M (0.0395266)") -> ("pm_hat_opt"=w1792:dbl[])  [unwired: 1 in, 1 out]
                  }
                  frame True {
                    # "Use current optimal point as initial guess for next iteration"
                    n168 = mathscript code="pm_init = pm_init';\ny_meas = y_meas*1e-4;  % convert from Gauss to Tesla\nn_par = length(pm_init);\niteration = 0;  % current number of \nstop = 0;  % stop flag\nMaxIter = 100;   % maximum number of iteration\nepsilon_1 = 1e-10;  % convergence tolerance for gradient\nepsilon_2 = 1e-9;  % convergence tolerance for parameter\nepsilon_3 = 1e-15;  % convergence tolerance for residual error\nepsilon_4 = 1e-8;  % determines acceptance of a L-M step\npm = pm_init; % initialization on parameters\nlambda_0 = 1e-3;  % user-specified initial lambda\n% Jacobian initialization\nJ = Analytic_Jacobian_Mag_cir_array_test(pm_init,xyz_s,meas_dir_s);\n% initialize L-M parameters\nlambda = lambda_0*max(diag(J'*J));\nv = 2;  % scale factor\nwhile ( ~stop)\n    iteration = iteration + 1;\n    B_meas = PM_forward_field(pm,xyz_s,meas_dir_s);\n% compute residual error between model and measurement\n    err = (y_meas - B_meas)';\n    if ( norm(err)^2< epsilon_3 &&  iteration > 2 )\n        stop = 1;\n        break;\n    end\n    % compute gradient\n    grad = J'*err;\n    % check stopping criterion 1\n    if ( max(abs(grad)) < epsilon_1  &&  iteration > 2 )\n        stop = 1;\n        break\n    end\n    % parameter increment change\n    delta = (J'*J + lambda*eye(n_par))\\J'*err;  % simplest version\n    % check stopping criterion 2 \n    if ( max(abs(delta)./(abs(pm)+1e-20)) < epsilon_2  &&  iteration > 2 )\n        stop = 1;\n        break\n    end\n    pm_try = pm + delta;\n    % evaluate value using pm_try\n    B_meas_try = PM_forward_field(pm_try,xyz_s,meas_dir_s);  % compute measurement based on given direction\n    err_try = (y_meas - B_meas_try)';\n    % compute rho for determining acceptance\n    rho = (err'*err - err_try'*err_try)/(delta'*(lambda*delta + J'*err) );\n    if rho > epsilon_4   % if better\n        pm = pm_try;  % accpet pm_try\n        lambda = lambda*max( 1/3, 1-(2*rho-1)^3 );\n        v = 2;\n             % update Jacobian matrix\n        J = Analytic_Jacobian_Mag_cir_array_test(pm,xyz_s,meas_dir_s);\n    else      % if not better\n        lambda = lambda*v;\n        v = 2*v;\n    end\n    if ( iteration == MaxIter )\n        stop = 1;\n    end\nend\n\npm_hat_opt = pm;"("meas_dir_s"=w2757, "xyz_s"=w2758, "y_meas"=w2761, "pm_init"=w2759) -> ("pm_hat_opt"=w2760:dbl[])  [unwired: 1 in, 1 out]
                  }
                }
                "pm_hat_opt" <- w1790
              }
            }
            n169 = Subtract(x=w1536, y=w1535) -> (x-y=→"Sensing time":u32)
          }
        }
        n170 = flat-sequence {
          frame #0 {
            n171 = xnode "Digital output (1 sample) 2"("C/DIO6 (DIO6)"="Reset Actuation") -> ()  [unwired: 1 in, 1 out]
            n172 = xnode "Digital output (1 sample) 3"("C/DIO7 (DIO7)"="Reset Feeding") -> ()  [unwired: 1 in, 1 out]
          }
        }
      }
    }
    frame #2 {
      n173 = xnode "PWM 3"("Duty Cycle"=0.0) -> ()  [unwired: 1 in, 1 out]
    }
  }
